vi "Main_NoAndor.vi"() -> ()   [LabVIEW 2014]
doc: "This is the main user interface of the Raman spectroscopy system."
uses:
  C:/Users/light/Desktop/Chuanzhen/Labview/Raman/dll/Thorlabs.MotionControl.Controls.dll
  dll/Thorlabs.MotionControl.Controls.dll
  TypeDef/States.ctl
  TypeDef/StageDeviceOut.ctl
  TypeDef/StageHandleIn.ctl
  <vilib>/Utility/miscctls.llb/LVPoint32TypeDef.ctl
  TypeDef/LaserSpot.ctl
  TypeDef/GalvoInput.ctl
  C:/Users/light/Desktop/Chuanzhen/Labview/Raman/dll/ThorLabs.MotionControl.KCube.DCServoCLI.dll
  dll/ThorLabs.MotionControl.KCube.DCServoCLI.dll
  TypeDef/StageSelect.ctl
  TypeDef/inputImages.ctl
  C:/Users/light/Desktop/Chuanzhen/Labview/Raman/dll/Thorlabs.MotionControl.GenericMotorCLI.dll
  dll/Thorlabs.MotionControl.GenericMotorCLI.dll
panel:
  in  "a2":dbl caption="Offset"
  out "Spot Y":dbl
  out "Spot X":dbl
  in  "Box":cluster{"Width":dbl, " Height":dbl}={"Width"=200.0, " Height"=214.0}
  in  "Galvo Reset":bool
  in  "a1":dbl=8.2 caption="Offset"
  in  "a0":dbl=4.0 caption="Offset"
  in  "Galvo Stop":bool
  out "Total_Frame_Y":dbl
  out "Total_Frame_X":dbl
  out "Frame_Y":dbl
  out "Frame_X":dbl
  in  "Destination":dbl=12.0
  in  "Save Path":path=path "C:/Users/light/Desktop/Chuanzhen/test"
  in  "Scan":bool
  in  "Velocity: X and Y axis":T1(radio)=enum."0.05mm"
  in  "MoveTo":bool
  in  "Jogstep of Z axis":T2(radio)=enum."10step"
  in  "Z axis_d":bool
  in  "Z axis_u":bool
  in  "Y axis_F":bool
  in  "Y axis_B":bool
  out "Y_axis":dbl
  out "X_axis":dbl
  out "Z_axis":dbl
  in  "Reset":bool
  in  "X axis_L":bool
  in  "X axis_R":bool
  in  "Down":bool
  in  "Top":bool
  in  "Right":bool
  in  "Left":bool
  in  "Snap":bool
  out "Boolean":bool
  in  "Pixel Size Y (um)":dbl=0.0877
  in  "LaserSpot":bool
  in  "Pixel Size X (um)":dbl=0.0877
  in  "Aim":bool
  in  "Galvo DC":bool
  out "Sample Rate":dbl=1000.0 format="%0.2f"
  out "Initialization finished":bool
  out "Focal plane (mm)":dbl
  out "Delay (s)":dbl=0.9 format="%#_13g"
  in  "Jog size (um)":dbl=2.0
  out "ZoomRatio":dbl format="%#_2g"
  in  "Focus":bool
  out "Live video":picture caption="600 x 480"
  in  "Next step":bool
  in  "Camera ID":u32
  out "Bits/Pixel":i32=8
  in  "Autogain":bool
  in  "Master Gain":i32(slide) min=0 max=100 scale=0.0..100.0
  in  "Hotpixel correction 2":bool
  in  "Blacklevel compensation":bool
  in  "Edge Filter":i32(ring)=2 items=["High"=1, "Low"=2]
  in  "Edge Filter Enable / Disable":bool
  in  "Exposure time (ms)":dbl(slide)=11.094175438596492 min=0.008982456140350877 max=101.68743859649123 step=0.05487719298245614 scale=0.008982456140350877..101.68743859649123 scale format="%#.3g"
  in  "Pixel clock":i32(slide)=20 min=7 max=86 scale=7.0..86.0
  in  "Frame rate":dbl(slide)=9.827169720568149 min=0.5 max=17.288905497022668 step=5.487719298245614e-05 scale=0.5..17.288905497022668 scale format="%^#_3g"
  in  "Blacklevel Offset":i32(slide) min=0 max=255 scale=0.0..255.0
  out "FPS":dbl=6.258409738085552
  out "Width":i32=640
  out "Height":i32=480
  in  "Stage Control":enum32{"X axis", "Y axis", "Z axis"}(tab)
  in  "X axis":refnum<k24>(container)
  in  "Y axis":refnum<k24>(container)
  in  "Z axis":refnum<k24>(container)
  in  "Quit":bool
  out "Waveform Graph":waveform(dbl)[](graph)=[{"t0"=timestamp(0 s since 1904-01-01), "dt"=0.001, "Y"=[]}]
  # "Camera Control"
  # "Galvo Control"
  # "Objective: CFI Plan Fluor ELWD 60x (1.27 NA) \nThe depth of field: 1.78 um\nPixel Size: 0.0877um/px"
  # "Attention: \ndon't click button very fast"
  # "Auto Focus"
  # "Aim"
  # "Motor Control"
  # "Adjust laser spot lightly"
  # "Stage Scan"
  # "Total_Frame"
  # "Current_Frame"
  # "X"
  # "Y"
  # "Focus distance ia about 2mm"
  # "Stepsize:"
  # "Jogstep:"
  # "0.00003mm/step"
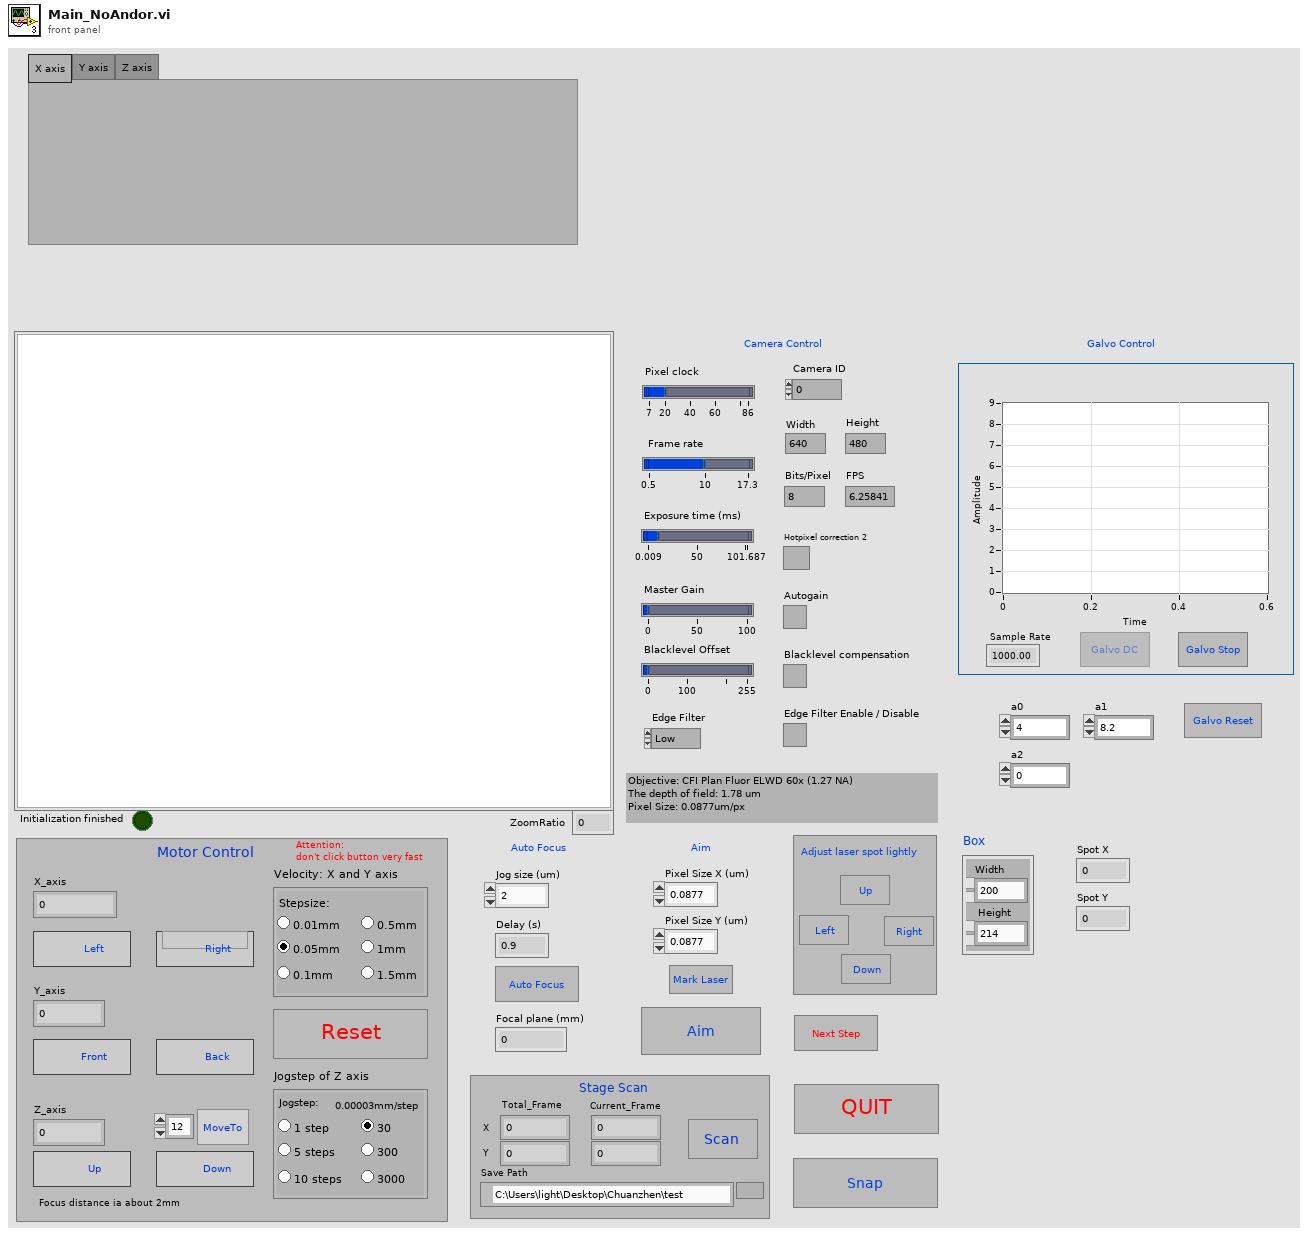
[diagram p1: front panel]
types:
  T1 = enum32{"0.01mm", "0.05mm", "0.1mm", "0.5mm", "1mm", "1.5mm"}
  T2 = enum32{"1step", "2step", "5step", "10step", "15step", "20step"}
  T3 = typedef "LaserSpot.ctl" = cluster{"Laser X":dbl, "Laser Y":dbl}
  T4 = cluster{"left":i16, "top":i16, "right":i16, "bottom":i16}
  T5 = typedef "LVPoint32TypeDef.ctl" = cluster{"Horizontal":i32, "Vertical":i32}
  T6 = typedef "StageHandleIn.ctl" = cluster{"Z StageHandle in":refnum<k24>, "X StageHandle in":refnum<k24>, "Y StageHandle in":refnum<k24>}
  T7 = typedef "StageDeviceOut.ctl" = cluster{"Device Z":refnum<k24>, "Device X":refnum<k24>, "Device Y":refnum<k24>}
  T8 = typedef "States.ctl" = enum16{"Initialize", "CMOS live", "Shut down"}
  T9 = enum8{"Enabled", "Disabled", "Disabled and Grayed Out"}
  T10 = typedef "GalvoInput.ctl" = cluster{"Sample Rate":dbl, "Sample Clock Source":tag, "Max Voltage":dbl, "Min Voltage":dbl, "Physical Channel(s)":tag}
  T11 = cluster{"Width":u16, "Style":enum32{"Solid", "Dash", "Dot", "DashDot", "DashDotDot"}}
  T12 = typedef "StageSelect.ctl" = enum16{"X axis", "Y axis", "Z axis"}
  T13 = typedef "inputImages.ctl" = cluster{"Image2":u8[][], "Image3":u8[][], "Image4":u8[][], "Image1":u8[][]}
  T14 = typedef "StageHandleOut.ctl" = cluster{"Z StageHandle out":refnum<k24>, "X StageHandle out":refnum<k24>, "Y StageHandle out":refnum<k24>}
  T15 = typedef "LVBoundsTypeDef.ctl" = cluster{"Width":u32, "Height":u32}
  T16 = typedef "imagedata.ctl" = cluster{"image type":i32, "image depth":i32, "image":u8[], "mask":u8[], "colors":u32[], "Rectangle":cluster{"left":i16, "top":i16, "right":i16, "bottom":i16}}
  T17 = typedef "LVPositionTypeDef.ctl" = cluster{"Left":i32, "Top":i32}
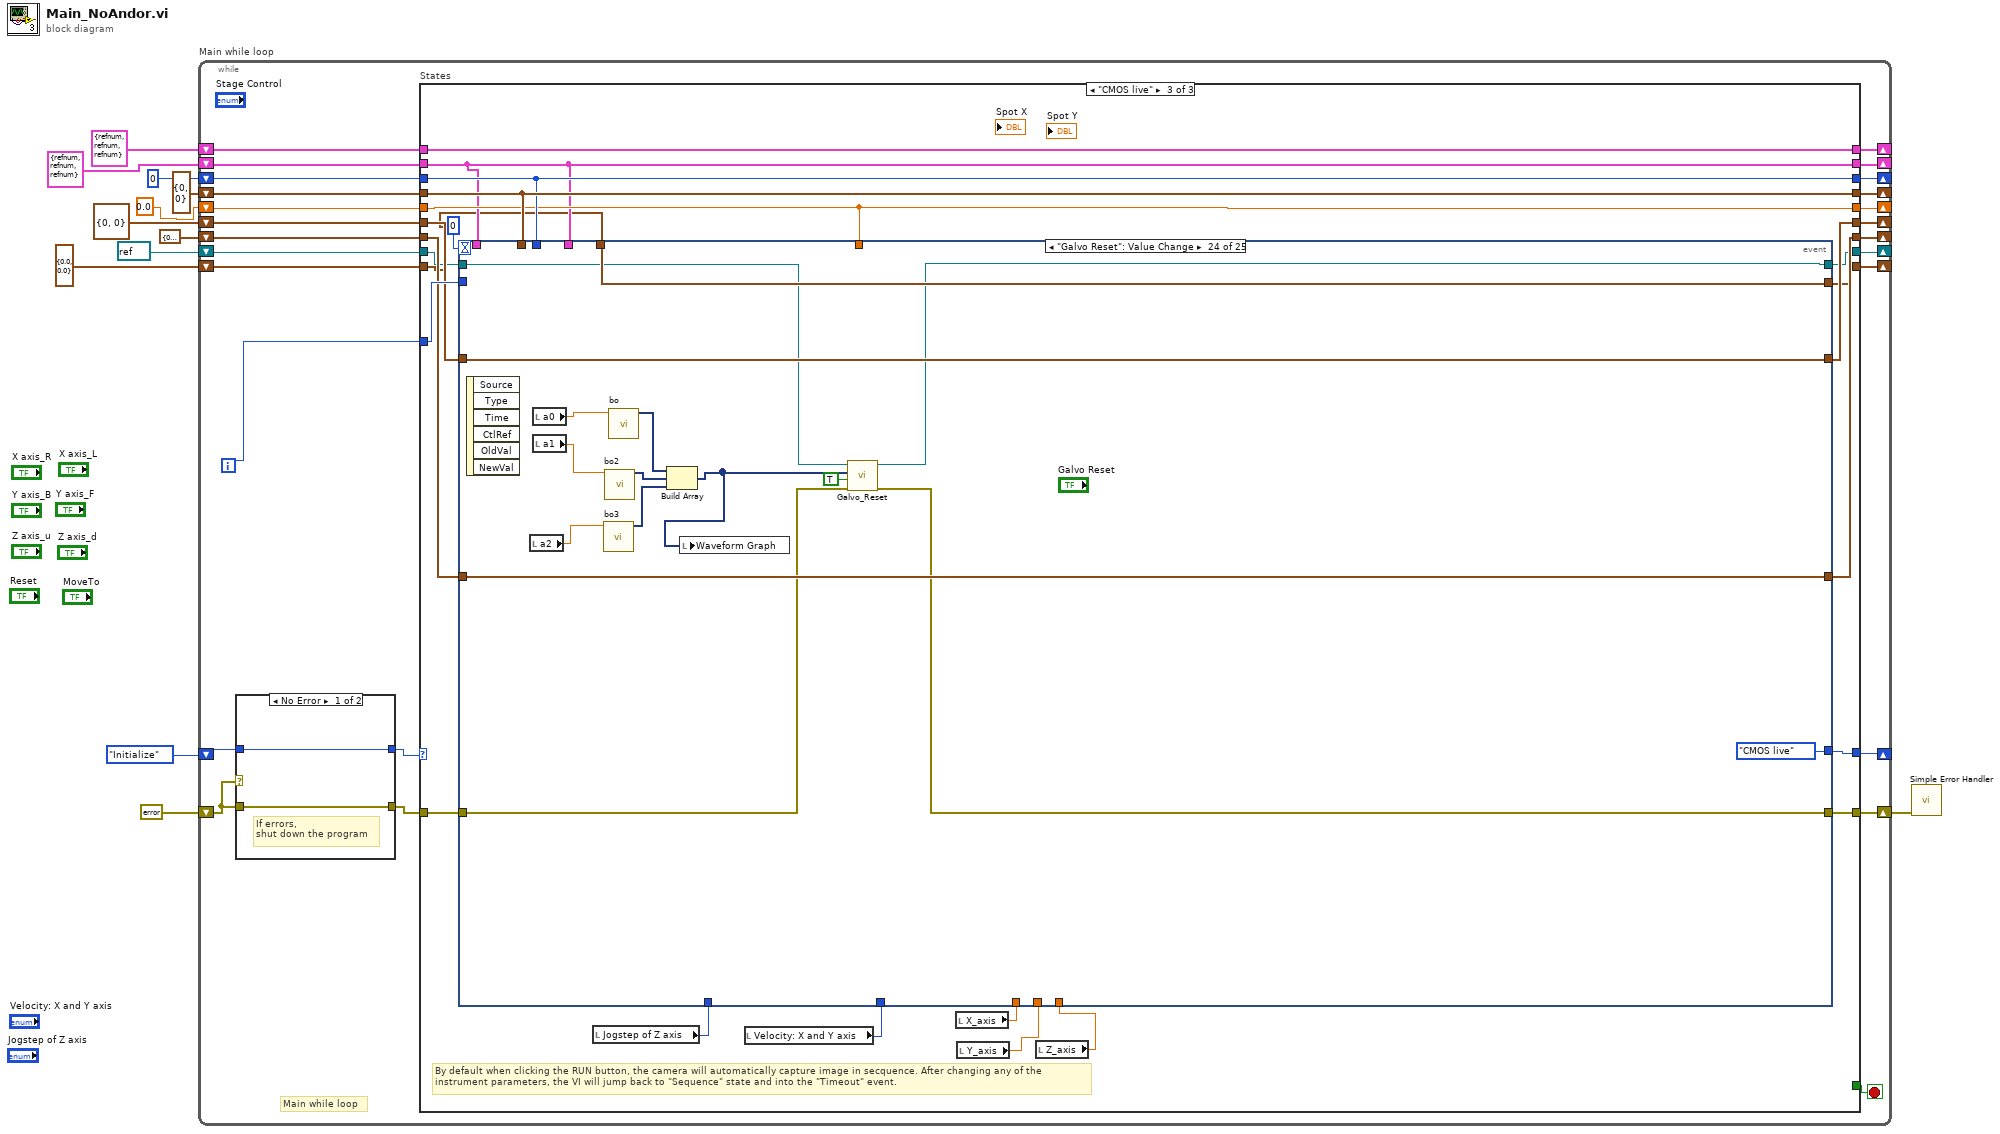
[diagram p0: block diagram]
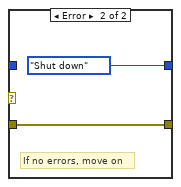
[diagram p2: hidden frame]
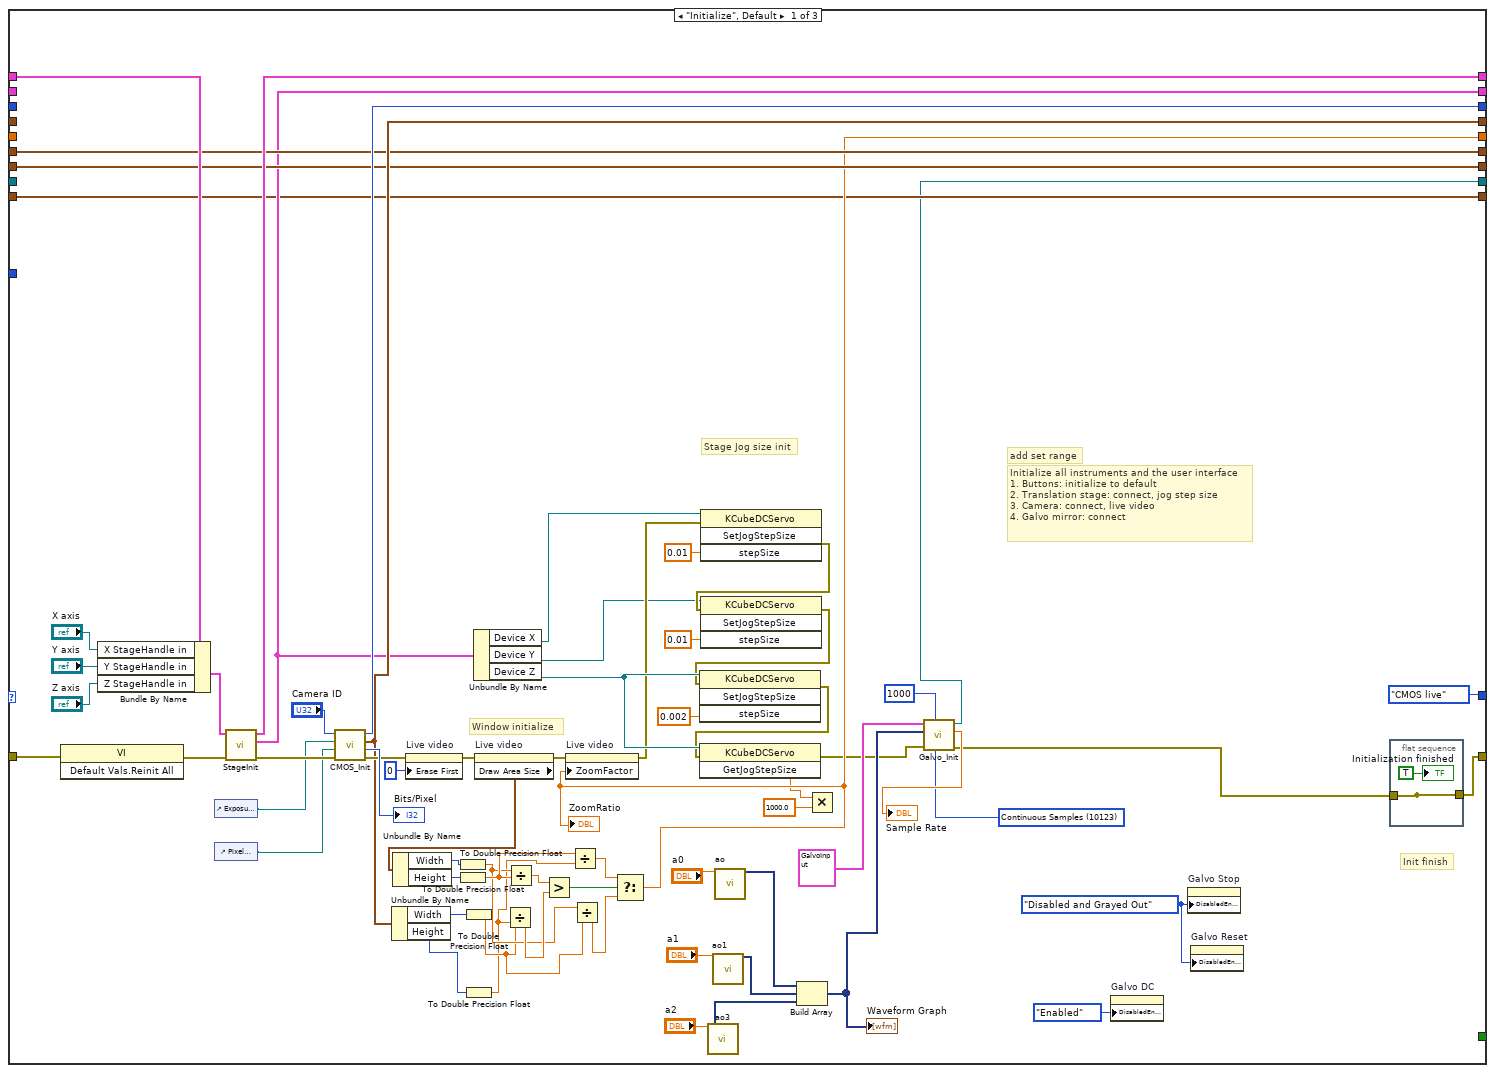
[diagram p3: hidden frame]
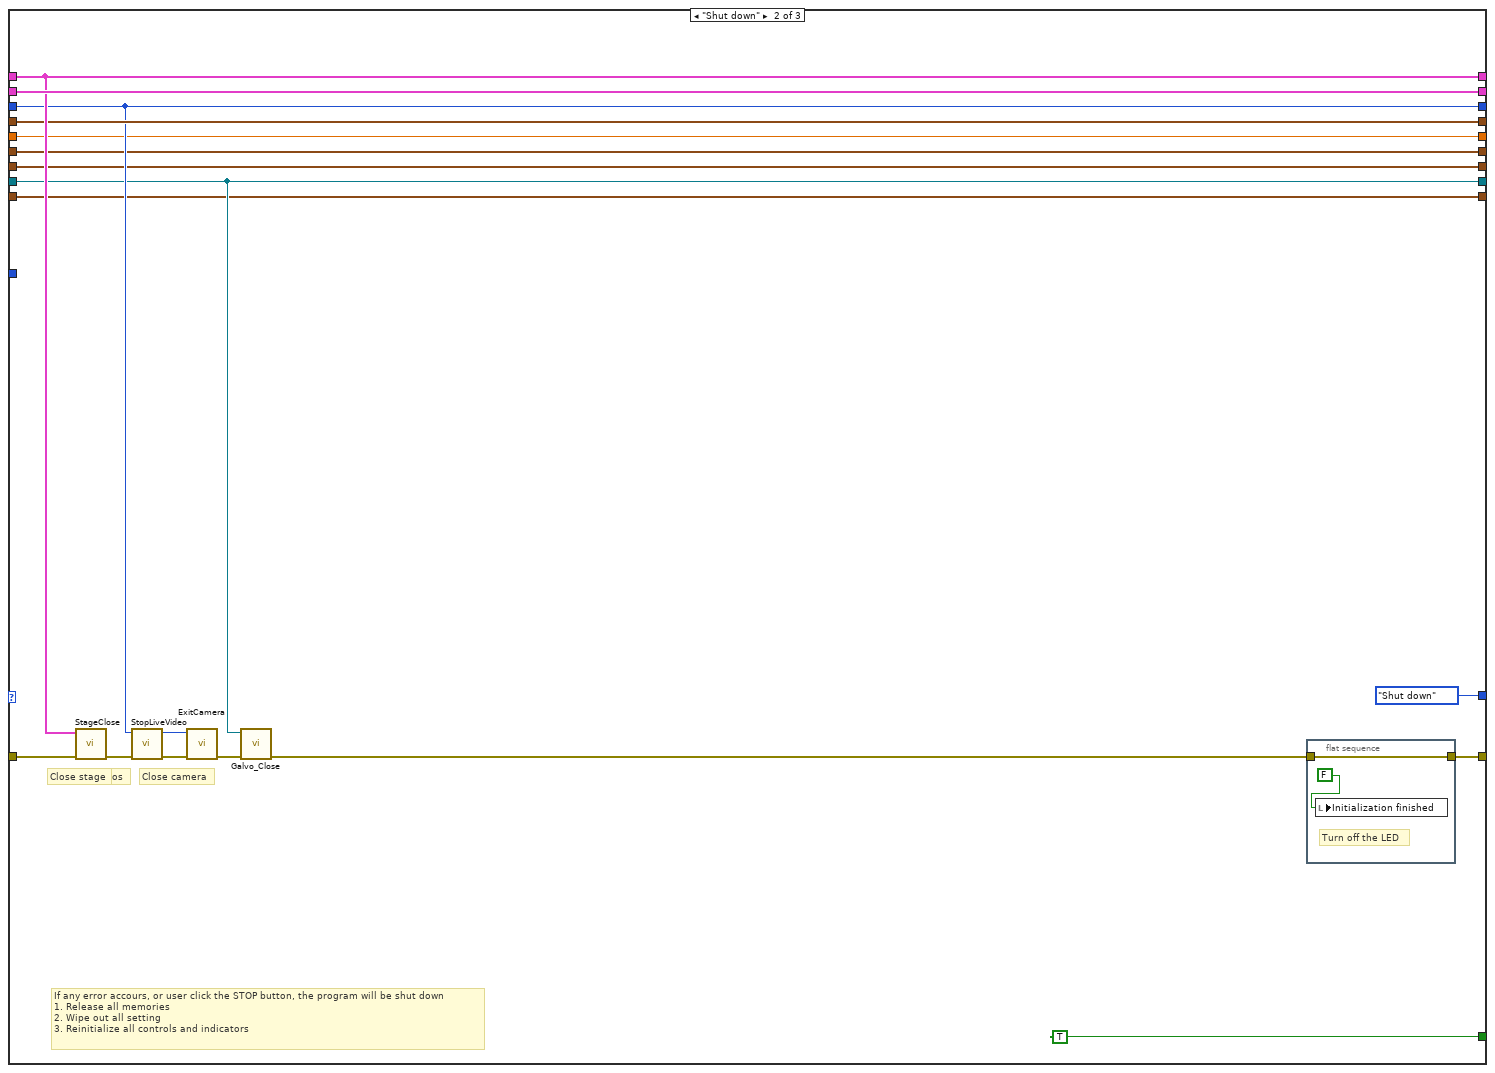
[diagram p4: hidden frame]
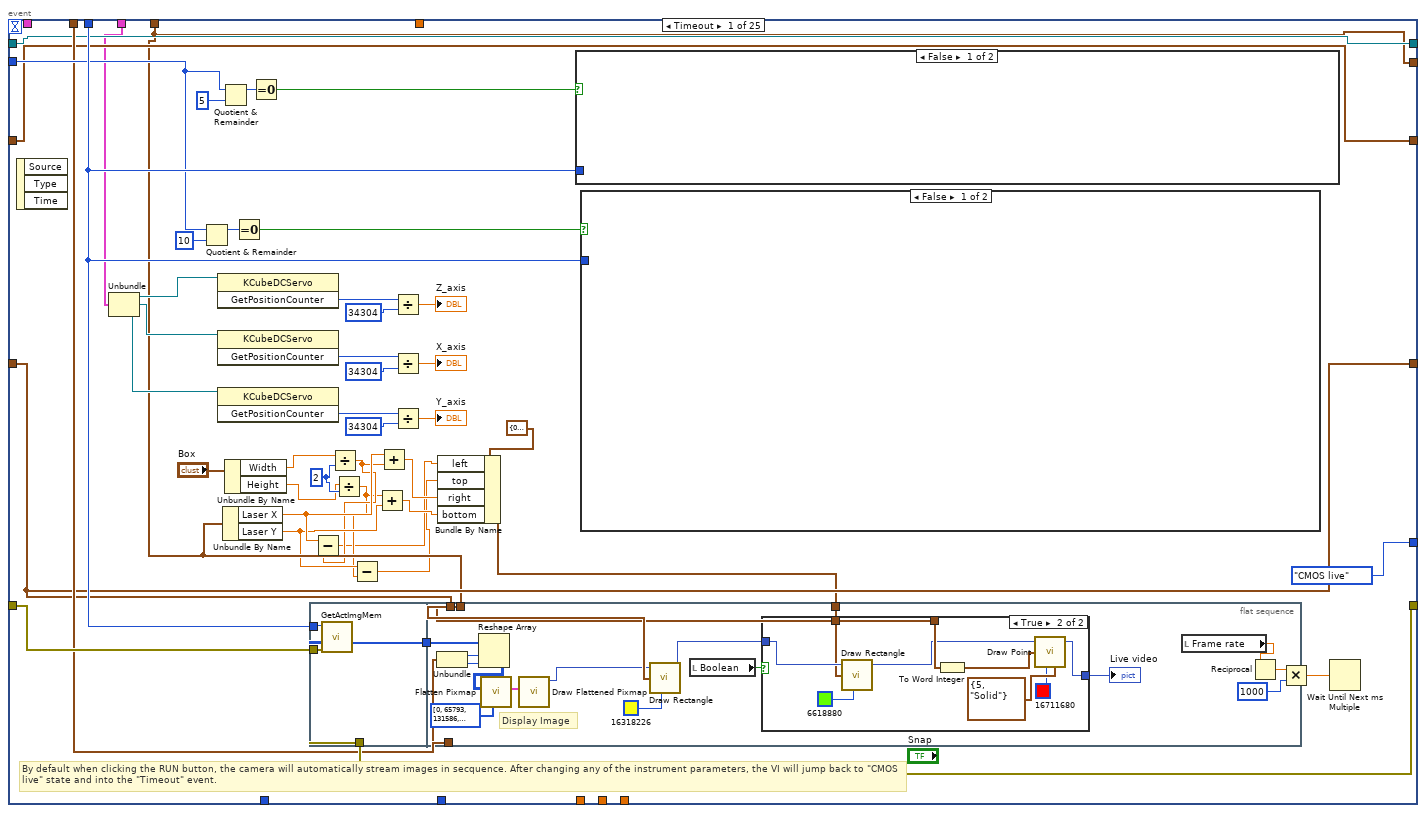
[diagram p5: hidden frame]
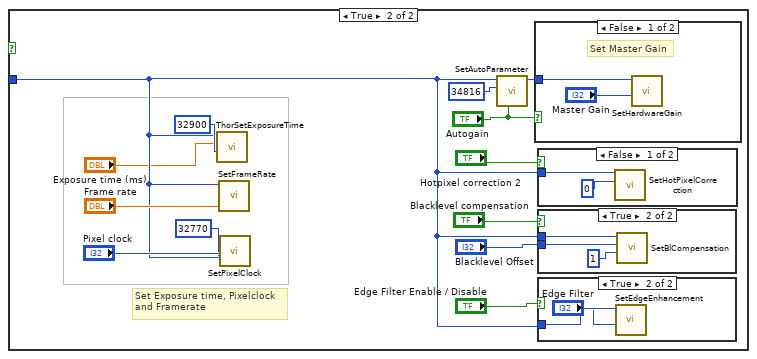
[diagram p6: hidden frame]
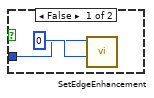
[diagram p7: hidden frame]
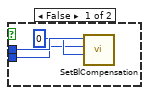
[diagram p8: hidden frame]
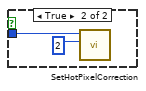
[diagram p9: hidden frame]
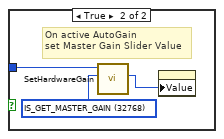
[diagram p10: hidden frame]
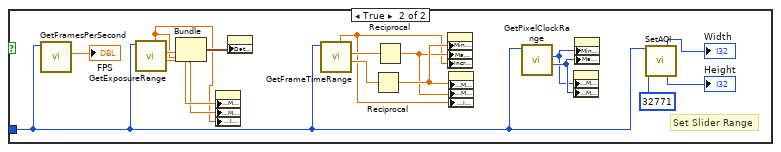
[diagram p11: hidden frame]
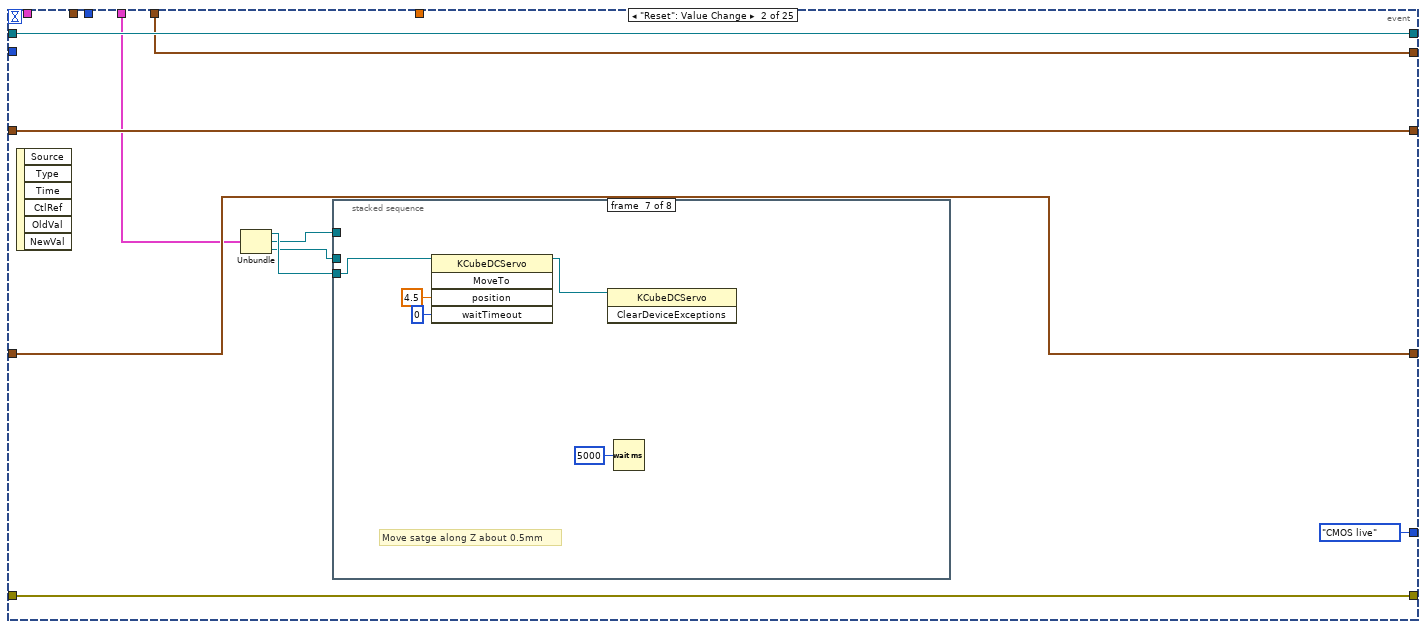
[diagram p13: hidden frame]
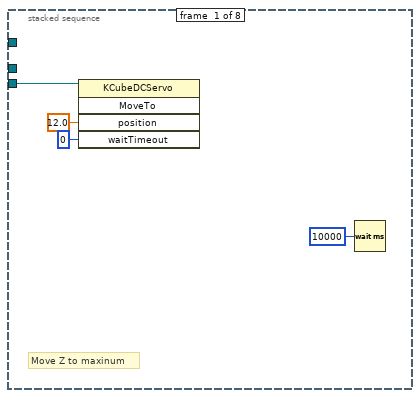
[diagram p14: hidden frame]
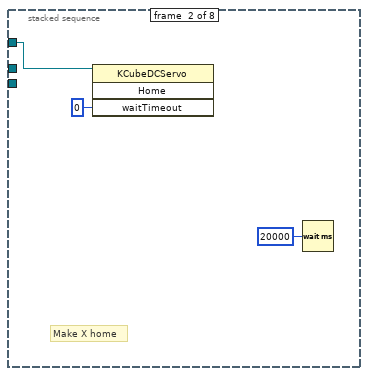
[diagram p15: hidden frame]
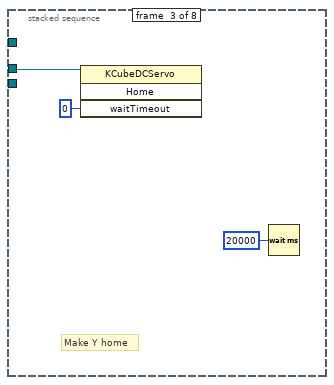
[diagram p16: hidden frame]
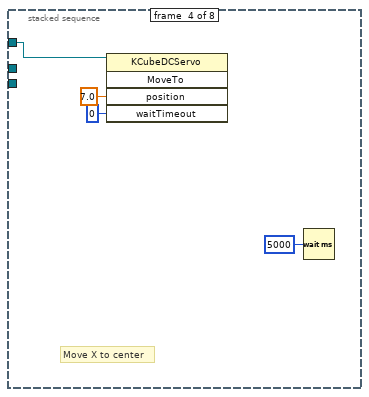
[diagram p17: hidden frame]
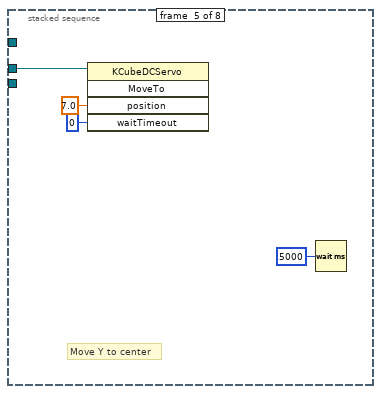
[diagram p18: hidden frame]
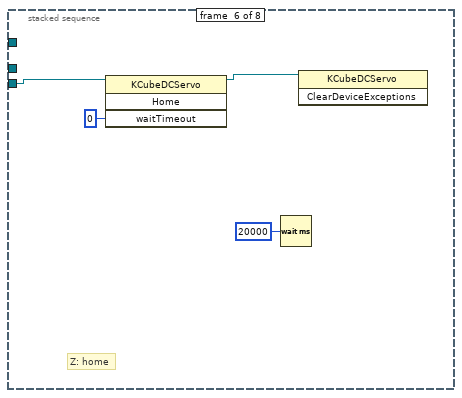
[diagram p19: hidden frame]
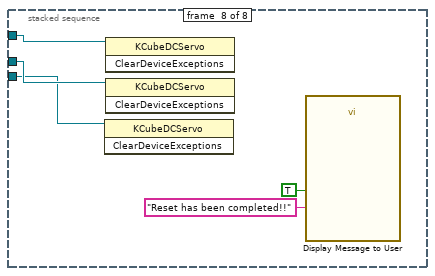
[diagram p20: hidden frame]
diagram:
  n1 = while "Main while loop" {
    shift-right: [w33] -> _
    shift-left: States."Initialize" -> [w38]
    shift-right: [w36] -> w10
    shift-left: errorcluster {"status"=FALSE, "code"=0, "source"=""} ("error out") -> [w32]
    shift-right: [w30] -> _
    shift-left: T6 {"Z StageHandle in"=refnum, "X StageHandle in"=refnum, "Y StageHandle in"=refnum} ("StageHandle In") -> [w31]
    shift-right: [w29] -> _
    shift-left: T7 {"Device Z"=refnum, "Device X"=refnum, "Device Y"=refnum} ("Device Out") -> [w28]
    shift-right: [w27] -> _
    shift-left: u32 0 ("CMOS Handle Out") -> [w26]
    shift-right: [w24] -> _
    shift-left: cluster{"Height":i32, "Width":i32} {"Height"=0, "Width"=0} ("WidthAndHeight") -> [w23]
    shift-right: [w22] -> _
    shift-left: 0.0 -> [w17]
    shift-right: [w21] -> _
    shift-left: T5 {"Horizontal"=0, "Vertical"=0} ("Coords") -> [w20]
    shift-right: [w19] -> _
    shift-left: T4 {"left"=0, "top"=0, "right"=0, "bottom"=0} ("rect") -> [w18]
    shift-right: [w16] -> _
    shift-left: refnum<k21> refnum ("task out") -> [w15]
    shift-right: [w14] -> _
    shift-left: T3 {"Laser X"=0.0, "Laser Y"=0.0} ("LaserSpot 2") -> [w13]
    i -> [w25]
    stop <- w34 stop-if-true
    # "Main while loop"
    n2 = case shown="No Error" w32 {
      tunnel: w32 -> [w40 w42]
      tunnel: [w40 w42] -> w35
      tunnel: w38 -> [w39 _]
      tunnel: [w39 States."Shut down"] -> w37
      frame No Error {
        # "If errors,\nshut down the program"
      }
      frame Error {
        # "If no errors, move on"
      }
    }
    n3 = case "States" shown="\"CMOS live\"" w37 {
      tunnel: [w53 w117 w152] -> w36
      tunnel: w35 -> [w109 w127 w153]
      tunnel: [_ TRUE _] -> w34
      tunnel: [States."CMOS live" States."Shut down" w154] -> w33
      tunnel: w31 -> [w107 w126 w155]
      tunnel: [w106 w126 w155] -> w30
      tunnel: [w73 w128 w142] -> w29
      tunnel: w28 -> [_ w128 w142]
      tunnel: [w100 w121 w148] -> w27
      tunnel: w26 -> [_ w121 w148]
      tunnel: w25 -> [_ _ w150]
      tunnel: [w81 w125 w149] -> w24
      tunnel: w23 -> [_ w125 w149]
      tunnel: [w74 w120 w143] -> w22
      tunnel: w17 -> [_ w120 w143]
      tunnel: [w76 w119 w147] -> w21
      tunnel: w20 -> [w76 w119 w146]
      tunnel: [w75 w118 w145] -> w19
      tunnel: w18 -> [w75 w118 w144]
      tunnel: [w54 w115 w140] -> w16
      tunnel: w15 -> [_ w115 w141]
      tunnel: [w59 w113 w139] -> w14
      tunnel: w13 -> [w59 w113 w138]
      frame "Initialize", Default {
        w45 = 10123 items=["Finite Samples"=10178, "Continuous Samples"=10123, "Hardware Timed Single Point"=12522] ("Sample Mode")
        w47 = T9."Disabled and Grayed Out" ("Disabled")
        # "Init finish"
        # "add set range"
        # "Stage Jog size init"
        # "Window initialize"
        # "Initialize all instruments and the user interface\n1. Buttons: initialize to default\n2. Translation stage: connect, jog step size\n3. Camera: connect, live video\n4. Galvo mirror: connect"
        n4 = invoke class="VI" method="Default Vals.Reinit All"(error in=w109) -> (error out=w108:errorcluster)  [unwired: 2 in, 2 out]
        n5 = Bundle By Name(cluster=w107, "X StageHandle in"="X axis", "Y StageHandle in"="Y axis", "Z StageHandle in"="Z axis") -> (w105:T6)
        n6 = control-ref of="Exposure time (ms)"() -> (w99:refnum<vi>)
        n7 = control-ref of="Pixel clock"() -> (w98:refnum<vi>)
        n8 = call "StageInit.vi"("error in (no error)"=w108, "StageHandle In"=w105) -> ("error out"=w101:errorcluster, "Device Out"=w73:T7, "StageHandle Out"=w106:T14)  [unwired: 7 in]
        n9 = call "CMOS_Init.vi"("error in"=w101, "Pixel clock"=w98, "Exposure time"=w99, "Camera ID"="Camera ID") -> ("error out"=w95:errorcluster, "Bits/Pixel"=→"Bits/Pixel":i32, "WidthAndHeight"=w81:cluster{"Height":i32, "Width":i32}, "CMOS Handle Out"=w100:u32)  [unwired: 3 in]
        n10 = Unbundle By Name(w81) -> ("Width"=w80:i32, "Height"=w79:i32)
        n11 = property on="Live video" class="Pict"(error in=w95, "Erase First"=u8 0) -> (error out=w83:errorcluster)  [unwired: 1 in, 1 out]
        n12 = To Double Precision Float(number=w80) -> (double precision float=w78:dbl)
        n13 = To Double Precision Float(number=w79) -> (double precision float=w77:dbl)
        n14 = Unbundle By Name(w73) -> ("Device X"=w62:refnum<k24>, "Device Y"=w61:refnum<k24>, "Device Z"=w71:refnum<k24>)
        n15 = property on="Live video" class="Pict"(error in=w83) -> (error out=w82:errorcluster, "Draw Area Size"=w93:T15)  [unwired: 1 in, 1 out]
        n16 = Unbundle By Name(w93) -> ("Width"=w91:u32, "Height"=w92:u32)
        n17 = To Double Precision Float(number=w91) -> (double precision float=w85:dbl)
        n18 = To Double Precision Float(number=w92) -> (double precision float=w87:dbl)
        n19 = Divide(x=w78, y=w77) -> (x/y=w88:dbl)
        n20 = Divide(x=w85, y=w87) -> (x/y=w90:dbl)
        n21 = Greater?(x=w90, y=w88) -> (0:w89:bool)
        n22 = Divide(x=w87, y=w77) -> (x/y=w86:dbl)
        n23 = Divide(x=w85, y=w78) -> (x/y=w84:dbl)
        n24 = Select(t=w86, s=w89, f=w84) -> (s? t:f=w74:dbl)
        "ZoomRatio" <- w74
        n25 = property on="Live video" class="Pict"(error in=w82, "ZoomFactor"=w74) -> (error out=w65:errorcluster)  [unwired: 1 in, 1 out]
        n26 = invoke class="KCubeDCServo" method="SetJogStepSize"(reference=w62, error in=w65, "stepSize"=0.01) -> (error out=w64:errorcluster)  [unwired: 1 in, 3 out]
        n27 = invoke class="KCubeDCServo" method="SetJogStepSize"(reference=w61, error in=w64, "stepSize"=0.01) -> (error out=w63:errorcluster)  [unwired: 1 in, 3 out]
        n28 = invoke class="KCubeDCServo" method="SetJogStepSize"(reference=w71, error in=w63, "stepSize"=0.002) -> (error out=w70:errorcluster)  [unwired: 1 in, 3 out]
        n29 = invoke class="KCubeDCServo" method="GetJogStepSize"(reference=w71, error in=w70) -> (error out=w56:errorcluster, "GetJogStepSize"=w69:dbl)  [unwired: 1 in, 1 out]
        n30 = call "ao3"("Offset"="a2") -> ("DC"=w60:dynamicdata)  [unwired: 13 in, 1 out]
        n31 = call "ao1"("Offset"="a1") -> ("DC"=w50:dynamicdata)  [unwired: 13 in, 1 out]
        n32 = call "ao"("Offset"="a0") -> ("DC"=w49:dynamicdata)  [unwired: 13 in, 1 out]
        n33 = Build Array(w49, w50, w60) -> (w57:dynamicdata[])
        "Waveform Graph" <- w57
        n34 = Multiply(x=w69, y=1000.0) -> ()  [unwired: 1 out]
        n35 = call "Galvo_Init.vi"("Sample Mode"=w45, "samples per channel"=1000, "error in"=w56, "Signal array"=w57, "Galvo_Input"=T10 {"Sample Rate"=1000.0, "Sample Clock Source"="OnboardClock", "Max Voltage"=10.0, "Min Voltage"=-10.0, "Physical Channel(s)"="Dev1/ao0,Dev1/ao1,Dev1/ao3"} ("Galvo1_1")) -> ("error out"=w48:errorcluster, "Actual Sample Rate"=→"Sample Rate":dbl, "task out"=w54:refnum<k21>)  [unwired: 4 in]
        n36 = property on="Galvo DC" class="Bool"("DisabledEnum"=T9."Enabled" ("Disabled")) -> ()  [unwired: 2 in, 2 out]
        n37 = property on="Galvo Stop" class="Bool"("DisabledEnum"=w47) -> ()  [unwired: 2 in, 2 out]
        n38 = property on="Galvo Reset" class="Bool"("DisabledEnum"=w47) -> ()  [unwired: 2 in, 2 out]
        n39 = flat-sequence {
          tunnel: [w111] -> _
          tunnel: w48 -> [w111]
          tunnel: [w111] -> w53
          frame #0 {
            "Initialization finished" <- TRUE ("Initialization finished")
          }
        }
      }
      frame "Shut down" {
        # "Close 3 galvos"
        # "Close camera"
        # "Close stage"
        # "If any error accours, or user click the STOP button, the program will be shut down\n1. Release all memories\n2. Wipe out all setting\n3. Reinitialize all controls and indicators"
        n40 = call "StageClose.vi"("error in (no error)"=w127, "StageHandle In"=w126) -> ("error out"=w124:errorcluster)  [unwired: 9 in]
        n41 = call "StopLiveVideo.vi"("error in"=w124, "Camera Handle In"=w121) -> ("error out"=w123:errorcluster, "Camera Handle Out"=w122:u32)  [unwired: 8 in]
        n42 = call "ExitCamera.vi"("error in"=w123, "Camera Handle In"=w122) -> ("error out"=w116:errorcluster)  [unwired: 9 in]
        n43 = call "Galvo_Close.vi"("error in"=w116, "task/channels in"=w115) -> ("error out"=w114:errorcluster)  [unwired: 9 in]
        n44 = flat-sequence {
          tunnel: w114 -> [w132]
          tunnel: [w132] -> w117
          frame #0 {
            # "Turn off the LED"
            n45 = local write "Initialization finished"(FALSE ("Initialization finished")) -> ()
          }
        }
      }
      frame "CMOS live" {
        # "By default when clicking the RUN button, the camera will automatically capture image in secquence. After changing any of the \ninstrument parameters, the VI will jump back to \"Sequence\" state and into the \"Timeout\" event."
        n46 = local read "Jogstep of Z axis"() -> (w133:T2)
        n47 = local read "Velocity: X and Y axis"() -> (w137:T1)
        n48 = local read "X_axis"() -> (w136:dbl)
        n49 = local read "Y_axis"() -> (w135:dbl)
        n50 = local read "Z_axis"() -> (w134:dbl)
        n51 = event shown="[23] \"Galvo Reset\": Value Change" {
          selector: _ -> [_ _ _ _ _ _ _ _ _ _ _ _ _ _ _ _ _ _ _ _ _ _ _ _ _]
          dyn-events: _ -> [_ _ _ _ _ _ _ _ _ _ _ _ _ _ _ _ _ _ _ _ _ _ _ _ _]
          timeout: 0 -> [_ _ _ _ _ _ _ _ _ _ _ _ _ _ _ _ _ _ _ _ _ _ _ _ _]
          tunnel: [States."CMOS live" States."CMOS live" States."CMOS live" States."CMOS live" States."CMOS live" States."CMOS live" States."CMOS live" States."CMOS live" States."CMOS live" States."CMOS live" States."CMOS live" States."Shut down" States."CMOS live" States."CMOS live" States."Shut down" States."CMOS live" States."CMOS live" States."CMOS live" States."CMOS live" States."CMOS live" States."CMOS live" States."CMOS live" States."CMOS live" States."CMOS live" States."CMOS live"] -> w154
          tunnel: w153 -> [w192 w290 w328 w597 w620 w645 w668 w693 w717 w737 w738 w756 w760 w768 w800 w847 w917 w939 w950 w961 w972 w983 w988 w1003 w1013]
          tunnel: [w191 w290 w327 w597 w620 w645 w668 w693 w717 w737 w738 w756 w760 w768 w800 w819 w918 w939 w950 w961 w972 w983 w987 w1002 w1014] -> w152
          tunnel: w148 -> [w190 _ w326 _ _ _ _ _ _ _ w747 _ _ _ _ w844 _ _ _ _ _ _ _ _ _]
          tunnel: w150 -> [w189 _ _ _ _ _ _ _ _ _ _ _ _ _ _ _ _ _ _ _ _ _ _ _ _]
          tunnel: w149 -> [w188 _ w325 _ _ _ _ _ _ _ w740 _ _ _ _ w843 _ _ _ _ _ _ _ _ _]
          tunnel: [w186 w289 w337 w596 w619 w644 w667 w692 w716 w736 w751 w755 w762 w770 w799 w849 w921 w938 w949 w960 w971 w982 w993 w1009 w1019] -> w147
          tunnel: w146 -> [w186 w289 w337 w596 w619 w644 w667 w692 w716 w736 w751 w755 _ w770 w799 w849 w921 w938 w949 w960 w971 w982 w993 w1009 w1019]
          tunnel: [w187 w288 w323 w595 w618 w643 w666 w691 w715 w735 w750 w754 w761 w773 w798 w842 w916 w927 w948 w959 w970 w981 w992 w1008 w1018] -> w145
          tunnel: w144 -> [w187 w288 w323 w595 w618 w643 w666 w691 w715 w735 w750 w754 w761 _ w798 w842 w916 w927 w948 w959 w970 w981 w992 w1008 w1018]
          tunnel: w143 -> [_ _ _ _ _ _ _ _ _ _ _ _ _ w772 _ _ _ _ _ _ _ _ _ _ _]
          tunnel: w142 -> [_ _ _ _ _ _ _ _ _ _ _ _ _ _ _ w818 _ _ _ _ _ _ _ _ _]
          tunnel: w142 -> [w183 w284 w329 w592 w614 w637 w661 w684 w709 w728 _ _ _ _ _ w840 w905 _ _ _ _ _ _ _ _]
          tunnel: [w185 w287 w336 w594 w617 w642 w665 w690 w714 w734 w749 w753 w759 w767 w797 w803 w920 w937 w947 w958 w969 w980 w990 w1004 w1012] -> w140
          tunnel: w141 -> [w185 w287 w336 w594 w617 w642 w665 w690 w714 w734 w749 w753 w759 w767 w797 w803 w920 w937 w947 w958 w969 w980 w989 w1005 w1015]
          tunnel: [w168 w286 w334 w593 w616 w641 w664 w689 w713 w733 w748 w752 w758 w766 w796 w802 w882 w925 w944 w953 w965 w976 w986 w1007 w1017] -> w139
          tunnel: w138 -> [w168 w286 w334 w593 w616 w641 w664 w689 w713 w733 w748 w752 w758 w766 w796 w802 w882 _ w943 w954 w966 w977 w986 w1007 w1017]
          tunnel: w137 -> [_ _ _ w584 w609 w632 w657 _ _ _ _ _ _ _ _ _ _ _ _ _ _ _ _ _ _]
          tunnel: w136 -> [_ _ _ w587 w612 _ _ _ _ _ _ _ _ _ _ _ _ _ _ _ _ _ _ _ _]
          tunnel: w135 -> [_ _ _ _ _ w634 w659 _ _ _ _ _ _ _ _ _ _ _ _ _ _ _ _ _ _]
          tunnel: w134 -> [_ _ _ _ _ _ _ w681 w705 _ _ _ _ _ _ _ _ _ _ _ _ _ _ _ _]
          tunnel: w133 -> [_ _ _ _ _ _ _ w685 w708 _ _ _ _ _ _ _ _ _ _ _ _ _ _ _ _]
          event Timeout {
            w167 = 2
            # "By default when clicking the RUN button, the camera will automatically stream images in secquence. After changing any of the instrument parameters, the VI will jump back to \"CMOS live\" state and into the \"Timeout\" event."
            n52 = event-data() -> ()  [unwired: 1 in, 3 out]
            n53 = Unbundle(w183) -> ("Device Z"=w173:refnum<k24>, "Device X"=w172:refnum<k24>, "Device Y"=w171:refnum<k24>)
            n54 = Quotient & Remainder(x=w189, y=10) -> (x-y*floor(x/y)=w199:i32)  [unwired: 1 out]
            n55 = invoke class="KCubeDCServo" method="GetPositionCounter"(reference=w173) -> ("GetPositionCounter"=w182:i32)  [unwired: 2 in, 2 out]
            n56 = invoke class="KCubeDCServo" method="GetPositionCounter"(reference=w172) -> ("GetPositionCounter"=w181:i32)  [unwired: 2 in, 2 out]
            n57 = invoke class="KCubeDCServo" method="GetPositionCounter"(reference=w171) -> ("GetPositionCounter"=w180:i32)  [unwired: 2 in, 2 out]
            n58 = Quotient & Remainder(x=w189, y=5) -> (x-y*floor(x/y)=w202:i32)  [unwired: 1 out]
            n59 = Unbundle By Name(w168) -> ("Laser X"=w162:dbl, "Laser Y"=w161:dbl)
            n60 = Unbundle By Name("Box") -> ("Width"=w166:dbl, "Height"=w165:dbl)
            n61 = Equal To 0?(x=w199) -> (x = 0?=w197:bool)
            n62 = Equal To 0?(x=w202) -> (x = 0?=w201:bool)
            n63 = flat-sequence {
              tunnel: [w254] -> w203
              tunnel: w190 -> [w255]
              tunnel: w192 -> [w253]
              tunnel: [w252] -> w191
              tunnel: w203 -> [w270]
              tunnel: w188 -> [w269]
              tunnel: w187 -> [w262]
              tunnel: w168 -> [w258]
              tunnel: w156 -> [w256]
              frame #0 {
                n64 = call "GetActImgMem.vi"("error in"=w253, "Camera Handle In"=w255) -> ("error out"=w252:errorcluster, "Image Memory Out"=w254:u8[])  [unwired: 6 in, 2 out]
              }
              frame #1 {
                # "Display Image"
                n65 = Unbundle(w269) -> ("Height"=w268:i32, "Width"=w267:i32)
                n66 = Reshape Array(w270, w268, w267) -> (w266:u8[][])
                n67 = call <vilib>:"Flatten Pixmap.vi"("colors"=u32[] [0, 65793, 131586, 197379, 263172, 328965, 394758, 460551, 526344, 592137, 657930, 723723, 789516, 855309, 921102, 986895, 1052688, 1118481, 1184274, 1250067, 1315860, 1381653, 1447446, 1513239, 1579032, 1644825, 1710618, 1776411, 1842204, 1907997, 1973790, 2039583, 2105376, 2171169, 2236962, 2302755, 2368548, 2434341, 2500134, 2565927, 2631720, 2697513, 2763306, 2829099, 2894892, 2960685, 3026478, 3092271, 3158064, 3223857, 3289650, 3355443, 3421236, 3487029, 3552822, 3618615, 3684408, 3750201, 3815994, 3881787, 3947580, 4013373, 4079166, 4144959, 4210752, 4276545, 4342338, 4408131, 4473924, 4539717, 4605510, 4671303, 4737096, 4802889, 4868682, 4934475, 5000268, 5066061, 5131854, 5197647, 5263440, 5329233, 5395026, 5460819, 5526612, 5592405, 5658198, 5723991, 5789784, 5855577, 5921370, 5987163, 6052956, 6118749, 6184542, 6250335, 6316128, 6381921, 6447714, 6513507, 6579300, 6645093, 6710886, 6776679, 6842472, 6908265, 6974058, 7039851, 7105644, 7171437, 7237230, 7303023, 7368816, 7434609, 7500402, 7566195, 7631988, 7697781, 7763574, 7829367, 7895160, 7960953, 8026746, 8092539, 8158332, 8224125, 8289918, 8355711, 8421504, 8487297, 8553090, 8618883, 8684676, 8750469, 8816262, 8882055, 8947848, 9013641, 9079434, 9145227, 9211020, 9276813, 9342606, 9408399, 9474192, 9539985, 9605778, 9671571, 9737364, 9803157, 9868950, 9934743, 10000536, 10066329, 10132122, 10197915, 10263708, 10329501, 10395294, 10461087, 10526880, 10592673, 10658466, 10724259, 10790052, 10855845, 10921638, 10987431, 11053224, 11119017, 11184810, 11250603, 11316396, 11382189, 11447982, 11513775, 11579568, 11645361, 11711154, 11776947, 11842740, 11908533, 11974326, 12040119, 12105912, 12171705, 12237498, 12303291, 12369084, 12434877, 12500670, 12566463, 12632256, 12698049, 12763842, 12829635, 12895428, 12961221, 13027014, 13092807, 13158600, 13224393, 13290186, 13355979, 13421772, 13487565, 13553358, 13619151, 13684944, 13750737, 13816530, 13882323, 13948116, 14013909, 14079702, 14145495, 14211288, 14277081, 14342874, 14408667, 14474460, 14540253, 14606046, 14671839, 14737632, 14803425, 14869218, 14935011, 15000804, 15066597, 15132390, 15198183, 15263976, 15329769, 15395562, 15461355, 15527148, 15592941, 15658734, 15724527, 15790320, 15856113, 15921906, 15987699, 16053492, 16119285, 16185078, 16250871, 16316664, 16382457, 16448250, 16514043, 16579836, 16645629, 16711422, 0] ("output array 2"), "8-bit pixmap"=w266) -> ("image data"=w265:T16)  [unwired: 9 in]
                n68 = call <vilib>:"Draw Flattened Pixmap.vi"("image data"=w265) -> ("new picture"=w257:picture)  [unwired: 8 in]
                n69 = call <vilib>:"Draw Rectangle.vi"("picture"=w257, "rect"=w262, "color(black)"=u32 16318226) -> ("new picture"=w261:picture)  [unwired: 6 in]
                n70 = local read "Boolean"() -> (w259:bool)
                n71 = case shown="True" w259 {
                  tunnel: w261 -> [w271 w275]
                  tunnel: [w271 w277] -> w260
                  tunnel: w258 -> [_ w276]
                  tunnel: w256 -> [_ w273]
                  frame False {
                  }
                  frame True {
                    n72 = call <vilib>:"Draw Rectangle.vi"("picture"=w275, "rect"=w273, "color(black)"=u32 6618880) -> ("new picture"=w274:picture)  [unwired: 6 in]
                    n73 = To Word Integer(number=w276) -> (16bit integer=w278:cluster{"Laser X":i16, "Laser Y":i16})
                    n74 = call <vilib>:"Draw Point.vi"("picture"=w274, "point(x,y)"=w278, "color(black)"=u32 16711680, "pen"=T11 {"Width"=5, "Style"=enum."Solid"}) -> ("new picture"=w277:picture)  [unwired: 5 in]
                  }
                }
                "Live video" <- w260
              }
            }
            n75 = Divide(x=w166, y=w167) -> (x/y=w160:dbl)
            n76 = Subtract(x=w162, y=w160) -> (x-y=w158:dbl)
            n77 = Divide(x=w165, y=w167) -> (x/y=w159:dbl)
            n78 = Subtract(x=w161, y=w159) -> (x-y=w157:dbl)
            n79 = Add(x=w159, y=w161) -> (x+y=w163:dbl)
            n80 = Add(x=w162, y=w160) -> (x+y=w164:dbl)
            n81 = Divide(x=w182, y=34304) -> (x/y=→"Z_axis":dbl)
            n82 = Divide(x=w181, y=34304) -> (x/y=→"X_axis":dbl)
            n83 = Divide(x=w180, y=34304) -> (x/y=→"Y_axis":dbl)
            n84 = Bundle By Name(cluster=T4 {"left"=0, "top"=0, "right"=0, "bottom"=0} ("rect"), "left"=w158, "top"=w157, "right"=w164, "bottom"=w163) -> (w156:T4)
            n85 = case shown="False" w201 {
              tunnel: w190 -> [_ w238]
              frame False {
              }
              frame True {
                # "Set Slider Range"
                n86 = call "GetFramesPerSecond.vi"("Camera Handle In"=w238) -> ("FPS"=→"FPS":dbl)  [unwired: 8 in, 2 out]
                n87 = call "GetExposureRange.vi"("Camera Handle In"=w238) -> ("max"=w248:dbl, "min"=w249:dbl, "intervall"=w247:dbl)  [unwired: 6 in, 2 out]
                n88 = Bundle("min"=w249, "max"=w248, "intervall"=w247) -> (w250:cluster{"min":dbl, "max":dbl, "intervall":dbl})  [unwired: 1 in]
                n89 = property on="Exposure time (ms)" class="Schieberegler (strikt)"("Scale.Minimum"=w249, "Scale.Maximum"=w248, "Scale.Increment"=w247) -> ()  [unwired: 2 in, 2 out]
                n90 = property on="Exposure time (ms)" class="Schieberegler (strikt)"("Data Range"=w250) -> ()  [unwired: 2 in, 2 out]
                n91 = call "GetFrameTimeRange.vi"("Camera Handle In"=w238) -> ("max"=w244:dbl, "min"=w243:dbl, "interval"=w240:dbl)  [unwired: 6 in, 2 out]
                n92 = Reciprocal(x=w244) -> (1/x=w242:dbl)
                n93 = Reciprocal(x=w243) -> (1/x=w241:dbl)
                n94 = property on="Frame rate" class="Schieberegler (strikt)"("Minimum"=w242, "Maximum"=w241, "Increment"=w240) -> ()  [unwired: 2 in, 2 out]
                n95 = property on="Frame rate" class="Schieberegler (strikt)"("Scale.Minimum"=w242, "Scale.Maximum"=w241, "Scale.Increment"=w240) -> ()  [unwired: 2 in, 2 out]
                n96 = call "GetPixelClockRange.vi"("Camera Handle In"=w238) -> ("Max"=w246:i32, "Min"=w245:i32)  [unwired: 7 in, 2 out]
                n97 = property on="Pixel clock" class="Schieberegler (strikt)"("Scale.Minimum"=w245, "Scale.Maximum"=w246) -> ()  [unwired: 2 in, 2 out]
                n98 = property on="Pixel clock" class="Schieberegler (strikt)"("Minimum"=w245, "Maximum"=w246) -> ()  [unwired: 2 in, 2 out]
                n99 = call "SetAOI.vi"("Camera Handle In"=w238, "Mode"=32771) -> ("Width Out"=→"Width":i32, "Height Out"=→"Height":i32)  [unwired: 8 in, 4 out]
              }
            }
            n100 = case shown="False" w197 {
              tunnel: w190 -> [_ w207]
              frame False {
              }
              frame True {
                # "Set Exposure time, Pixelclock\nand Framerate"
                n101 = call "ThorSetExposureTime.vi"("Mode"=u16 32900, "Exposure Time"="Exposure time (ms)", "Camera Handle In"=w207) -> ()  [unwired: 6 in, 3 out]
                n102 = call "SetFrameRate.vi"("FPS"="Frame rate", "Camera Handle In"=w207) -> ()  [unwired: 7 in, 3 out]
                n103 = call "SetPixelClock.vi"("Mode"=32770, "Pixel Clock"="Pixel clock", "Camera Handle In"=w207) -> ()  [unwired: 6 in, 3 out]
                n104 = call "SetAutoParameter.vi"("enable"="Autogain", "Param"=34816, "Camera Handle In"=w207) -> ("Camera Handle Out"=w215:u32)  [unwired: 6 in, 2 out]
                n105 = case shown="False" "Autogain" {
                  tunnel: w215 -> [w231 w234]
                  frame False {
                    # "Set Master Gain"
                    n106 = call "SetHardwareGain.vi"("Master Gain"="Master Gain", "Camera Handle In"=w231) -> ()  [unwired: 7 in, 3 out]
                  }
                  frame True {
                    w233 = 32768 items=["IS_GET_MASTER_GAIN"=32768]
                    # "On active AutoGain\nset Master Gain Slider Value"
                    n107 = call "SetHardwareGain.vi"("Mode"=w233, "Camera Handle In"=w234) -> ("Value"=w235:i32)  [unwired: 7 in, 2 out]
                    n108 = property on="Master Gain" class="Slide (strict)"("Value"=w235) -> ()  [unwired: 2 in, 2 out]
                  }
                }
                n109 = case shown="False" "Hotpixel correction 2" {
                  tunnel: w207 -> [w228 w230]
                  frame False {
                    n110 = call "SetHotPixelCorrection.vi"("Mode"=0, "Camera Handle In"=w228) -> ()  [unwired: 7 in, 3 out]
                  }
                  frame True {
                    n111 = call "SetHotPixelCorrection.vi"("Mode"=2, "Camera Handle In"=w230) -> ()  [unwired: 7 in, 3 out]
                  }
                }
                n112 = case shown="True" "Blacklevel compensation" {
                  tunnel: w207 -> [w223 w226]
                  tunnel: "Blacklevel Offset" -> [w221 w224]
                  frame False {
                    n113 = call "SetBlCompensation.vi"("Mode"=0, "offset"=w221, "Camera Handle In"=w223) -> ()  [unwired: 6 in, 3 out]
                  }
                  frame True {
                    n114 = call "SetBlCompensation.vi"("Mode"=1, "offset"=w224, "Camera Handle In"=w226) -> ()  [unwired: 6 in, 3 out]
                  }
                }
                n115 = case shown="True" "Edge Filter Enable / Disable" {
                  tunnel: w207 -> [w217 w220]
                  frame False {
                    n116 = call "SetEdgeEnhancement.vi"("Mode"=0, "Camera Handle In"=w217) -> ()  [unwired: 8 in, 2 out]
                  }
                  frame True {
                    n117 = call "SetEdgeEnhancement.vi"("Mode"="Edge Filter", "Camera Handle In"=w220) -> ()  [unwired: 8 in, 2 out]
                  }
                }
              }
            }
            n118 = local read "Frame rate"() -> (w196:dbl)
            n119 = Reciprocal(x=w196) -> (1/x=w195:dbl)
            n120 = Multiply(x=w195, y=1000) -> (x*y=w193:dbl)
            n121 = Wait Until Next ms Multiple(millisecond multiple=w193) -> ()  [unwired: 1 out]
          }
          event "Reset": Value Change {
            n122 = event-data() -> ()  [unwired: 1 in, 6 out]
            n123 = Unbundle(w284) -> ("Device Z"=w283:refnum<k24>, "Device X"=w282:refnum<k24>, "Device Y"=w281:refnum<k24>)
            n124 = stacked-sequence {
              tunnel: w283 -> [w294 _ _ _ _ w312 w317 w318]
              tunnel: w281 -> [_ _ w298 _ w308 _ _ w319]
              tunnel: w282 -> [_ w295 _ w304 _ _ _ w320]
              frame #0 {
                # "Move Z to maxinum"
                n125 = invoke class="KCubeDCServo" method="MoveTo"(reference=w294, "position"=12.0, "waitTimeout"=0) -> ()  [unwired: 2 in, 5 out]
                n126 = Wait (ms)(milliseconds to wait=u32 10000) -> ()  [unwired: 1 out]
              }
              frame #1 {
                # "Make X home"
                n127 = invoke class="KCubeDCServo" method="Home"(reference=w295, "waitTimeout"=0) -> ()  [unwired: 2 in, 4 out]
                n128 = Wait (ms)(milliseconds to wait=u32 20000) -> ()  [unwired: 1 out]
              }
              frame #2 {
                # "Make Y home"
                n129 = invoke class="KCubeDCServo" method="Home"(reference=w298, "waitTimeout"=0) -> ()  [unwired: 2 in, 4 out]
                n130 = Wait (ms)(milliseconds to wait=u32 20000) -> ()  [unwired: 1 out]
              }
              frame #3 {
                # "Move X to center"
                n131 = invoke class="KCubeDCServo" method="MoveTo"(reference=w304, "position"=7.0, "waitTimeout"=0) -> ()  [unwired: 2 in, 5 out]
                n132 = Wait (ms)(milliseconds to wait=u32 5000) -> ()  [unwired: 1 out]
              }
              frame #4 {
                # "Move Y to center"
                n133 = invoke class="KCubeDCServo" method="MoveTo"(reference=w308, "position"=7.0, "waitTimeout"=0) -> ()  [unwired: 2 in, 5 out]
                n134 = Wait (ms)(milliseconds to wait=u32 5000) -> ()  [unwired: 1 out]
              }
              frame #5 {
                # "Z: home"
                n135 = invoke class="KCubeDCServo" method="Home"(reference=w312, "waitTimeout"=0) -> (reference out=w309:refnum<k24>)  [unwired: 2 in, 3 out]
                n136 = Wait (ms)(milliseconds to wait=u32 20000) -> ()  [unwired: 1 out]
                n137 = invoke class="KCubeDCServo" method="ClearDeviceExceptions"(reference=w309) -> ()  [unwired: 2 in, 3 out]
              }
              frame #6 {
                # "Move satge along Z about 0.5mm"
                n138 = invoke class="KCubeDCServo" method="MoveTo"(reference=w317, "position"=4.5, "waitTimeout"=0) -> (reference out=w313:refnum<k24>)  [unwired: 2 in, 4 out]
                n139 = invoke class="KCubeDCServo" method="ClearDeviceExceptions"(reference=w313) -> ()  [unwired: 2 in, 3 out]
                n140 = Wait (ms)(milliseconds to wait=u32 5000) -> ()  [unwired: 1 out]
              }
              frame #7 {
                n141 = invoke class="KCubeDCServo" method="ClearDeviceExceptions"(reference=w318) -> ()  [unwired: 2 in, 3 out]
                n142 = invoke class="KCubeDCServo" method="ClearDeviceExceptions"(reference=w320) -> ()  [unwired: 2 in, 3 out]
                n143 = invoke class="KCubeDCServo" method="ClearDeviceExceptions"(reference=w319) -> ()  [unwired: 2 in, 3 out]
                n144 = call "Display Message to User"("Enable"=TRUE, "Message"="Reset has been completed!!") -> ()  [unwired: 8 in, 2 out]
              }
            }
          }
          event "Scan": Value Change {
            n145 = event-data() -> ()  [unwired: 1 in, 6 out]
            n146 = Unbundle By Name(w323) -> ("left"=w333:i16, "top"=w331:i16, "right"=w332:i16, "bottom"=w330:i16)
            n147 = stacked-sequence {
              tunnel: w334 -> [_ w370 _ _]
              tunnel: w333 -> [_ w352 w403 _]
              tunnel: w332 -> [_ _ w404 _]
              tunnel: w331 -> [_ w351 w396 _]
              tunnel: w330 -> [_ _ w397 _]
              tunnel: w329 -> [_ w355 w395 _]
              tunnel: w328 -> [_ w354 _ _]
              tunnel: [_ w353 _ _] -> w327
              tunnel: w326 -> [w338 _ w394 _]
              tunnel: w325 -> [w339 _ w393 _]
              tunnel: "Save Path" -> [w341 _ w392 _]
              frame #0 {
                n148 = Unbundle(w339) -> ("Height"=w344:i32, "Width"=w343:i32)
                n149 = Build Path(base path=w341, name or relative path="Crop_Area.png") -> (appended path=w345:path)
                n150 = call "GetActImgMem.vi"("Camera Handle In"=w338) -> ("Image Memory Out"=w348:u8[])  [unwired: 7 in, 3 out]
                n151 = Reshape Array(w348, w344, w343) -> (w349:u8[][])
                n152 = call <vilib>:"Flatten Pixmap.vi"("colors"=u32[] [0, 65793, 131586, 197379, 263172, 328965, 394758, 460551, 526344, 592137, 657930, 723723, 789516, 855309, 921102, 986895, 1052688, 1118481, 1184274, 1250067, 1315860, 1381653, 1447446, 1513239, 1579032, 1644825, 1710618, 1776411, 1842204, 1907997, 1973790, 2039583, 2105376, 2171169, 2236962, 2302755, 2368548, 2434341, 2500134, 2565927, 2631720, 2697513, 2763306, 2829099, 2894892, 2960685, 3026478, 3092271, 3158064, 3223857, 3289650, 3355443, 3421236, 3487029, 3552822, 3618615, 3684408, 3750201, 3815994, 3881787, 3947580, 4013373, 4079166, 4144959, 4210752, 4276545, 4342338, 4408131, 4473924, 4539717, 4605510, 4671303, 4737096, 4802889, 4868682, 4934475, 5000268, 5066061, 5131854, 5197647, 5263440, 5329233, 5395026, 5460819, 5526612, 5592405, 5658198, 5723991, 5789784, 5855577, 5921370, 5987163, 6052956, 6118749, 6184542, 6250335, 6316128, 6381921, 6447714, 6513507, 6579300, 6645093, 6710886, 6776679, 6842472, 6908265, 6974058, 7039851, 7105644, 7171437, 7237230, 7303023, 7368816, 7434609, 7500402, 7566195, 7631988, 7697781, 7763574, 7829367, 7895160, 7960953, 8026746, 8092539, 8158332, 8224125, 8289918, 8355711, 8421504, 8487297, 8553090, 8618883, 8684676, 8750469, 8816262, 8882055, 8947848, 9013641, 9079434, 9145227, 9211020, 9276813, 9342606, 9408399, 9474192, 9539985, 9605778, 9671571, 9737364, 9803157, 9868950, 9934743, 10000536, 10066329, 10132122, 10197915, 10263708, 10329501, 10395294, 10461087, 10526880, 10592673, 10658466, 10724259, 10790052, 10855845, 10921638, 10987431, 11053224, 11119017, 11184810, 11250603, 11316396, 11382189, 11447982, 11513775, 11579568, 11645361, 11711154, 11776947, 11842740, 11908533, 11974326, 12040119, 12105912, 12171705, 12237498, 12303291, 12369084, 12434877, 12500670, 12566463, 12632256, 12698049, 12763842, 12829635, 12895428, 12961221, 13027014, 13092807, 13158600, 13224393, 13290186, 13355979, 13421772, 13487565, 13553358, 13619151, 13684944, 13750737, 13816530, 13882323, 13948116, 14013909, 14079702, 14145495, 14211288, 14277081, 14342874, 14408667, 14474460, 14540253, 14606046, 14671839, 14737632, 14803425, 14869218, 14935011, 15000804, 15066597, 15132390, 15198183, 15263976, 15329769, 15395562, 15461355, 15527148, 15592941, 15658734, 15724527, 15790320, 15856113, 15921906, 15987699, 16053492, 16119285, 16185078, 16250871, 16316664, 16382457, 16448250, 16514043, 16579836, 16645629, 16711422, 0] ("output array 2"), "8-bit pixmap"=w349) -> ("image data"=w346:T16)  [unwired: 9 in]
                n153 = Wait (ms)(milliseconds to wait=u32 300) -> ()  [unwired: 1 out]
                n154 = call <vilib>:"Write PNG File.vi"("image data"=w346, "path to PNG file"=w345) -> ()  [unwired: 8 in, 2 out]
              }
              frame #1 {
                n155 = Unbundle By Name(w370) -> ("Laser X"=w362:dbl, "Laser Y"=w361:dbl)
                n156 = Subtract(x=w362, y=w352) -> (x-y=w360:dbl)
                n157 = Subtract(x=w361, y=w351) -> (x-y=w358:dbl)
                n158 = Divide(x=0.0877, y=1000.0) -> (x/y=w359:dbl)
                n159 = Multiply(x=w359, y=w360) -> (x*y=w357:dbl)
                n160 = Multiply(x=w359, y=w358) -> (x*y=w356:dbl)
                n161 = call "StageReadPos.vi"("error in (no error)"=w354, "Stage Select"=StageSelect."X axis", "Device In"=w355) -> ("error out"=w369:errorcluster, "CurrentPosition"=w367:dbl)  [unwired: 7 in]
                n162 = call "StageReadPos.vi"("error in (no error)"=w354, "Stage Select"=StageSelect."Y axis", "Device In"=w355) -> ("error out"=w365:errorcluster, "CurrentPosition"=w364:dbl)  [unwired: 7 in]
                n163 = stacked-sequence {
                  tunnel: w369 -> [w389 _]
                  tunnel: w367 -> [w387 _]
                  tunnel: [w385 _] -> w363
                  tunnel: w357 -> [w384 _]
                  tunnel: w355 -> [w383 _]
                  frame #0 {
                    n164 = Add(x=w384, y=w387) -> (x+y=w386:dbl)
                    n165 = call "StageToPos.vi"("error in (no error)"=w389, "Move to pos"=w386, "Stage Select"=StageSelect."X axis", "Device In"=w383) -> ("error out"=w385:errorcluster)  [unwired: 7 in]
                  }
                  frame #1 {
                    n166 = Wait (ms)(milliseconds to wait=u32 400) -> ()  [unwired: 1 out]
                  }
                }
                n167 = stacked-sequence {
                  tunnel: w365 -> [w380 _]
                  tunnel: w364 -> [w379 _]
                  tunnel: w363 -> [w377 _]
                  tunnel: w356 -> [w375 _]
                  tunnel: w355 -> [w374 _]
                  tunnel: [w373 _] -> w353
                  frame #0 {
                    n168 = Add(x=w375, y=w379) -> (x+y=w378:dbl)
                    n169 = call "StageToPos.vi"("error in (no error)"=w380, "Move to pos"=w378, "Stage Select"=StageSelect."Y axis", "Device In"=w374) -> ("error out"=w376:errorcluster)  [unwired: 7 in]
                    n170 = Merge Errors(w377, w376) -> (w373:errorcluster)
                  }
                  frame #1 {
                    n171 = Wait (ms)(milliseconds to wait=u32 400) -> ()  [unwired: 1 out]
                  }
                }
                n172 = Wait (ms)(milliseconds to wait=u32 100) -> ()  [unwired: 1 out]
              }
              frame #2 {
                n173 = Subtract(x=w397, y=w396) -> (x-y=w399:i16)
                n174 = Subtract(x=w404, y=w403) -> (x-y=w402:i16)
                n175 = Divide(x=w399, y=i16 50) -> (x/y=w391:dbl)
                n176 = Divide(x=w402, y=i16 50) -> (x/y=w400:dbl)
                n177 = for {
                  N: w391 -> [w411]
                  tunnel: w400 -> [w405]
                  tunnel: w395 -> [w415]
                  tunnel: w394 -> [w414]
                  tunnel: w393 -> [w413]
                  tunnel: w392 -> [w412]
                  i -> [w408]
                  n178 = Round Toward -Infinity(1:w405) -> (0:→"Total_Frame_X":dbl)
                  n179 = Increment(x=w408) -> (x+1=→"Frame_Y":i32)
                  n180 = Divide(x=w408, y=2) -> (x/y=w420:dbl)
                  n181 = Round Toward -Infinity(1:w420) -> (0:w417:dbl)
                  n182 = Round Toward +Infinity(x=w420) -> (ceil(x): smallest int >= x=w418:dbl)
                  n183 = Equal?(x=w418, y=w417) -> (x = y?=w416:bool)
                  n184 = stacked-sequence {
                    tunnel: w416 -> [_ w433 w485]
                    tunnel: w405 -> [_ _ w484]
                    tunnel: w415 -> [w430 _ w483]
                    tunnel: w414 -> [_ w434 w482]
                    tunnel: w413 -> [_ w435 w481]
                    tunnel: w412 -> [_ w436 w480]
                    tunnel: w408 -> [_ w432 w479]
                    tunnel: w405 -> [_ w431 w478]
                    tunnel: [_ _ w477] -> w410
                    frame #0 {
                      w428 = 1 items=["Forward"=1, "Backward"=2] ("direction")
                      n185 = Unbundle By Name(w430) -> ("Device Y"=w429:refnum<k24>)  [unwired: 2 out]
                      n186 = Divide(x=0.0877 ("y"), y=1000.0) -> (x/y=w421:dbl)
                      n187 = Multiply(x=50.0, y=w421) -> (x*y=w424:dbl)
                      n188 = invoke class="KCubeDCServo" method="MoveRelative"(reference=w429, "direction"=w428, "stepSize"=w424, "waitTimeout"=0) -> ()  [unwired: 2 in, 6 out]
                      n189 = Wait (ms)(milliseconds to wait=u32 300) -> ()  [unwired: 1 out]
                    }
                    frame #1 {
                      n190 = case shown="False" w433 {
                        tunnel: w436 -> [w443 w462]
                        tunnel: w435 -> [w441 w461]
                        tunnel: w434 -> [w442 w460]
                        tunnel: w432 -> [w439 w458]
                        tunnel: w431 -> [w438 _]
                        frame False {
                          n191 = Round Toward -Infinity(1:w438) -> (0:w437:dbl)
                          n192 = Increment(x=w439) -> (x+1=w444:i32)
                          n193 = Number To Decimal String(number=w437) -> (decimal integer string=w440:string)  [unwired: 1 in]
                          n194 = Number To Decimal String(number=w444) -> (decimal integer string=w449:string)  [unwired: 1 in]
                          n195 = Concatenate Strings("x" ("string"), w440, "_y" ("string"), w449, ".png" ("string")) -> (w453:string)
                          n196 = Unbundle(w441) -> ("Height"=w447:i32, "Width"=w446:i32)
                          n197 = Build Path(base path=w443, name or relative path=w453) -> (appended path=w448:path)
                          n198 = call "GetActImgMem.vi"("Camera Handle In"=w442) -> ("Image Memory Out"=w456:u8[])  [unwired: 7 in, 3 out]
                          n199 = Reshape Array(w456, w447, w446) -> (w457:u8[][])
                          n200 = call <vilib>:"Flatten Pixmap.vi"("colors"=u32[] [0, 65793, 131586, 197379, 263172, 328965, 394758, 460551, 526344, 592137, 657930, 723723, 789516, 855309, 921102, 986895, 1052688, 1118481, 1184274, 1250067, 1315860, 1381653, 1447446, 1513239, 1579032, 1644825, 1710618, 1776411, 1842204, 1907997, 1973790, 2039583, 2105376, 2171169, 2236962, 2302755, 2368548, 2434341, 2500134, 2565927, 2631720, 2697513, 2763306, 2829099, 2894892, 2960685, 3026478, 3092271, 3158064, 3223857, 3289650, 3355443, 3421236, 3487029, 3552822, 3618615, 3684408, 3750201, 3815994, 3881787, 3947580, 4013373, 4079166, 4144959, 4210752, 4276545, 4342338, 4408131, 4473924, 4539717, 4605510, 4671303, 4737096, 4802889, 4868682, 4934475, 5000268, 5066061, 5131854, 5197647, 5263440, 5329233, 5395026, 5460819, 5526612, 5592405, 5658198, 5723991, 5789784, 5855577, 5921370, 5987163, 6052956, 6118749, 6184542, 6250335, 6316128, 6381921, 6447714, 6513507, 6579300, 6645093, 6710886, 6776679, 6842472, 6908265, 6974058, 7039851, 7105644, 7171437, 7237230, 7303023, 7368816, 7434609, 7500402, 7566195, 7631988, 7697781, 7763574, 7829367, 7895160, 7960953, 8026746, 8092539, 8158332, 8224125, 8289918, 8355711, 8421504, 8487297, 8553090, 8618883, 8684676, 8750469, 8816262, 8882055, 8947848, 9013641, 9079434, 9145227, 9211020, 9276813, 9342606, 9408399, 9474192, 9539985, 9605778, 9671571, 9737364, 9803157, 9868950, 9934743, 10000536, 10066329, 10132122, 10197915, 10263708, 10329501, 10395294, 10461087, 10526880, 10592673, 10658466, 10724259, 10790052, 10855845, 10921638, 10987431, 11053224, 11119017, 11184810, 11250603, 11316396, 11382189, 11447982, 11513775, 11579568, 11645361, 11711154, 11776947, 11842740, 11908533, 11974326, 12040119, 12105912, 12171705, 12237498, 12303291, 12369084, 12434877, 12500670, 12566463, 12632256, 12698049, 12763842, 12829635, 12895428, 12961221, 13027014, 13092807, 13158600, 13224393, 13290186, 13355979, 13421772, 13487565, 13553358, 13619151, 13684944, 13750737, 13816530, 13882323, 13948116, 14013909, 14079702, 14145495, 14211288, 14277081, 14342874, 14408667, 14474460, 14540253, 14606046, 14671839, 14737632, 14803425, 14869218, 14935011, 15000804, 15066597, 15132390, 15198183, 15263976, 15329769, 15395562, 15461355, 15527148, 15592941, 15658734, 15724527, 15790320, 15856113, 15921906, 15987699, 16053492, 16119285, 16185078, 16250871, 16316664, 16382457, 16448250, 16514043, 16579836, 16645629, 16711422, 0] ("output array 2"), "8-bit pixmap"=w457) -> ("image data"=w454:T16)  [unwired: 9 in]
                          n201 = Wait (ms)(milliseconds to wait=u32 300) -> ()  [unwired: 1 out]
                          n202 = call <vilib>:"Write PNG File.vi"("image data"=w454, "path to PNG file"=w448) -> ()  [unwired: 8 in, 2 out]
                        }
                        frame True {
                          n203 = Increment(x=w458) -> (x+1=w463:i32)
                          n204 = Number To Decimal String(number=w463) -> (decimal integer string=w468:string)  [unwired: 1 in]
                          n205 = Concatenate Strings("x" ("string"), "0" ("string"), "_y" ("string"), w468, ".png" ("string")) -> (w472:string)
                          n206 = Unbundle(w461) -> ("Height"=w466:i32, "Width"=w465:i32)
                          n207 = Build Path(base path=w462, name or relative path=w472) -> (appended path=w467:path)
                          n208 = call "GetActImgMem.vi"("Camera Handle In"=w460) -> ("Image Memory Out"=w475:u8[])  [unwired: 7 in, 3 out]
                          n209 = Reshape Array(w475, w466, w465) -> (w476:u8[][])
                          n210 = call <vilib>:"Flatten Pixmap.vi"("colors"=u32[] [0, 65793, 131586, 197379, 263172, 328965, 394758, 460551, 526344, 592137, 657930, 723723, 789516, 855309, 921102, 986895, 1052688, 1118481, 1184274, 1250067, 1315860, 1381653, 1447446, 1513239, 1579032, 1644825, 1710618, 1776411, 1842204, 1907997, 1973790, 2039583, 2105376, 2171169, 2236962, 2302755, 2368548, 2434341, 2500134, 2565927, 2631720, 2697513, 2763306, 2829099, 2894892, 2960685, 3026478, 3092271, 3158064, 3223857, 3289650, 3355443, 3421236, 3487029, 3552822, 3618615, 3684408, 3750201, 3815994, 3881787, 3947580, 4013373, 4079166, 4144959, 4210752, 4276545, 4342338, 4408131, 4473924, 4539717, 4605510, 4671303, 4737096, 4802889, 4868682, 4934475, 5000268, 5066061, 5131854, 5197647, 5263440, 5329233, 5395026, 5460819, 5526612, 5592405, 5658198, 5723991, 5789784, 5855577, 5921370, 5987163, 6052956, 6118749, 6184542, 6250335, 6316128, 6381921, 6447714, 6513507, 6579300, 6645093, 6710886, 6776679, 6842472, 6908265, 6974058, 7039851, 7105644, 7171437, 7237230, 7303023, 7368816, 7434609, 7500402, 7566195, 7631988, 7697781, 7763574, 7829367, 7895160, 7960953, 8026746, 8092539, 8158332, 8224125, 8289918, 8355711, 8421504, 8487297, 8553090, 8618883, 8684676, 8750469, 8816262, 8882055, 8947848, 9013641, 9079434, 9145227, 9211020, 9276813, 9342606, 9408399, 9474192, 9539985, 9605778, 9671571, 9737364, 9803157, 9868950, 9934743, 10000536, 10066329, 10132122, 10197915, 10263708, 10329501, 10395294, 10461087, 10526880, 10592673, 10658466, 10724259, 10790052, 10855845, 10921638, 10987431, 11053224, 11119017, 11184810, 11250603, 11316396, 11382189, 11447982, 11513775, 11579568, 11645361, 11711154, 11776947, 11842740, 11908533, 11974326, 12040119, 12105912, 12171705, 12237498, 12303291, 12369084, 12434877, 12500670, 12566463, 12632256, 12698049, 12763842, 12829635, 12895428, 12961221, 13027014, 13092807, 13158600, 13224393, 13290186, 13355979, 13421772, 13487565, 13553358, 13619151, 13684944, 13750737, 13816530, 13882323, 13948116, 14013909, 14079702, 14145495, 14211288, 14277081, 14342874, 14408667, 14474460, 14540253, 14606046, 14671839, 14737632, 14803425, 14869218, 14935011, 15000804, 15066597, 15132390, 15198183, 15263976, 15329769, 15395562, 15461355, 15527148, 15592941, 15658734, 15724527, 15790320, 15856113, 15921906, 15987699, 16053492, 16119285, 16185078, 16250871, 16316664, 16382457, 16448250, 16514043, 16579836, 16645629, 16711422, 0] ("output array 2"), "8-bit pixmap"=w476) -> ("image data"=w473:T16)  [unwired: 9 in]
                          n211 = Wait (ms)(milliseconds to wait=u32 300) -> ()  [unwired: 1 out]
                          n212 = call <vilib>:"Write PNG File.vi"("image data"=w473, "path to PNG file"=w467) -> ()  [unwired: 8 in, 2 out]
                        }
                      }
                    }
                    frame #2 {
                      n213 = case shown="False" w485 {
                        tunnel: w484 -> [w493 w542]
                        tunnel: w483 -> [w492 w541]
                        tunnel: w482 -> [w490 w540]
                        tunnel: w481 -> [w487 w539]
                        tunnel: w480 -> [w491 w538]
                        tunnel: w479 -> [w489 w537]
                        tunnel: w478 -> [w488 _]
                        tunnel: [w486 w536] -> w477
                        frame False {
                          n214 = for {
                            N: w493 -> [_]
                            tunnel: w492 -> [w500]
                            tunnel: w491 -> [w499]
                            tunnel: w490 -> [w498]
                            tunnel: w489 -> [w497]
                            tunnel: w488 -> [w496]
                            tunnel: w487 -> [w495]
                            tunnel: [w494] -> w486
                            i -> [w494]
                            n215 = stacked-sequence {
                              tunnel: w500 -> [_ w505 _]
                              tunnel: w499 -> [_ _ w524]
                              tunnel: w498 -> [_ _ w523]
                              tunnel: w497 -> [_ _ w518]
                              tunnel: w494 -> [_ _ w516]
                              tunnel: w496 -> [_ _ w515]
                              tunnel: w495 -> [_ _ w522]
                              frame #0 {
                                n216 = Wait (ms)(milliseconds to wait=u32 100) -> ()  [unwired: 1 out]
                              }
                              frame #1 {
                                w511 = 2 items=["Forward"=1, "Backward"=2] ("direction")
                                n217 = Unbundle By Name(w505) -> ("Device X"=w506:refnum<k24>)  [unwired: 2 out]
                                n218 = Divide(x=0.0877 ("y"), y=1000.0) -> (x/y=w503:dbl)
                                n219 = Multiply(x=50.0, y=w503) -> (x*y=w507:dbl)
                                n220 = invoke class="KCubeDCServo" method="MoveRelative"(reference=w506, "direction"=w511, "stepSize"=w507, "waitTimeout"=0) -> ()  [unwired: 2 in, 6 out]
                                n221 = Wait (ms)(milliseconds to wait=u32 450) -> ()  [unwired: 1 out]
                              }
                              frame #2 {
                                n222 = Round Toward -Infinity(1:w515) -> (0:w514:dbl)
                                n223 = Decrement(x=w514) -> (x-1=w513:dbl)
                                n224 = Subtract(x=w513, y=w516) -> (x-y=w512:dbl)
                                n225 = Increment(x=w518) -> (x+1=w517:i32)
                                n226 = Number To Decimal String(number=w512) -> (decimal integer string=w527:string)  [unwired: 1 in]
                                n227 = Number To Decimal String(number=w517) -> (decimal integer string=w526:string)  [unwired: 1 in]
                                n228 = Concatenate Strings("x" ("string"), w527, "_y" ("string"), w526, ".png" ("string")) -> (w531:string)
                                n229 = Unbundle(w522) -> ("Height"=w521:i32, "Width"=w520:i32)
                                n230 = Build Path(base path=w524, name or relative path=w531) -> (appended path=w525:path)
                                n231 = call "GetActImgMem.vi"("Camera Handle In"=w523) -> ("Image Memory Out"=w534:u8[])  [unwired: 7 in, 3 out]
                                n232 = Reshape Array(w534, w521, w520) -> (w535:u8[][])
                                n233 = call <vilib>:"Flatten Pixmap.vi"("colors"=u32[] [0, 65793, 131586, 197379, 263172, 328965, 394758, 460551, 526344, 592137, 657930, 723723, 789516, 855309, 921102, 986895, 1052688, 1118481, 1184274, 1250067, 1315860, 1381653, 1447446, 1513239, 1579032, 1644825, 1710618, 1776411, 1842204, 1907997, 1973790, 2039583, 2105376, 2171169, 2236962, 2302755, 2368548, 2434341, 2500134, 2565927, 2631720, 2697513, 2763306, 2829099, 2894892, 2960685, 3026478, 3092271, 3158064, 3223857, 3289650, 3355443, 3421236, 3487029, 3552822, 3618615, 3684408, 3750201, 3815994, 3881787, 3947580, 4013373, 4079166, 4144959, 4210752, 4276545, 4342338, 4408131, 4473924, 4539717, 4605510, 4671303, 4737096, 4802889, 4868682, 4934475, 5000268, 5066061, 5131854, 5197647, 5263440, 5329233, 5395026, 5460819, 5526612, 5592405, 5658198, 5723991, 5789784, 5855577, 5921370, 5987163, 6052956, 6118749, 6184542, 6250335, 6316128, 6381921, 6447714, 6513507, 6579300, 6645093, 6710886, 6776679, 6842472, 6908265, 6974058, 7039851, 7105644, 7171437, 7237230, 7303023, 7368816, 7434609, 7500402, 7566195, 7631988, 7697781, 7763574, 7829367, 7895160, 7960953, 8026746, 8092539, 8158332, 8224125, 8289918, 8355711, 8421504, 8487297, 8553090, 8618883, 8684676, 8750469, 8816262, 8882055, 8947848, 9013641, 9079434, 9145227, 9211020, 9276813, 9342606, 9408399, 9474192, 9539985, 9605778, 9671571, 9737364, 9803157, 9868950, 9934743, 10000536, 10066329, 10132122, 10197915, 10263708, 10329501, 10395294, 10461087, 10526880, 10592673, 10658466, 10724259, 10790052, 10855845, 10921638, 10987431, 11053224, 11119017, 11184810, 11250603, 11316396, 11382189, 11447982, 11513775, 11579568, 11645361, 11711154, 11776947, 11842740, 11908533, 11974326, 12040119, 12105912, 12171705, 12237498, 12303291, 12369084, 12434877, 12500670, 12566463, 12632256, 12698049, 12763842, 12829635, 12895428, 12961221, 13027014, 13092807, 13158600, 13224393, 13290186, 13355979, 13421772, 13487565, 13553358, 13619151, 13684944, 13750737, 13816530, 13882323, 13948116, 14013909, 14079702, 14145495, 14211288, 14277081, 14342874, 14408667, 14474460, 14540253, 14606046, 14671839, 14737632, 14803425, 14869218, 14935011, 15000804, 15066597, 15132390, 15198183, 15263976, 15329769, 15395562, 15461355, 15527148, 15592941, 15658734, 15724527, 15790320, 15856113, 15921906, 15987699, 16053492, 16119285, 16185078, 16250871, 16316664, 16382457, 16448250, 16514043, 16579836, 16645629, 16711422, 0] ("output array 2"), "8-bit pixmap"=w535) -> ("image data"=w532:T16)  [unwired: 9 in]
                                n234 = Wait (ms)(milliseconds to wait=u32 300) -> ()  [unwired: 1 out]
                                n235 = call <vilib>:"Write PNG File.vi"("image data"=w532, "path to PNG file"=w525) -> ()  [unwired: 8 in, 2 out]
                              }
                            }
                          }
                        }
                        frame True {
                          n236 = for {
                            N: w542 -> [_]
                            tunnel: w541 -> [w548]
                            tunnel: w540 -> [w547]
                            tunnel: w539 -> [w546]
                            tunnel: w538 -> [w545]
                            tunnel: w537 -> [w544]
                            tunnel: [w543] -> w536
                            i -> [w543]
                            n237 = stacked-sequence {
                              tunnel: w548 -> [_ w554 _]
                              tunnel: w547 -> [_ _ w574]
                              tunnel: w546 -> [_ _ w573]
                              tunnel: w545 -> [_ _ w571]
                              tunnel: w543 -> [_ _ w561]
                              tunnel: w544 -> [_ _ w563]
                              frame #0 {
                                n238 = Wait (ms)(milliseconds to wait=u32 100) -> ()  [unwired: 1 out]
                              }
                              frame #1 {
                                w559 = 1 items=["Forward"=1, "Backward"=2] ("direction")
                                n239 = Unbundle By Name(w554) -> ("Device X"=w553:refnum<k24>)  [unwired: 2 out]
                                n240 = Divide(x=0.0877 ("y"), y=1000.0) -> (x/y=w550:dbl)
                                n241 = Multiply(x=50.0, y=w550) -> (x*y=w555:dbl)
                                n242 = invoke class="KCubeDCServo" method="MoveRelative"(reference=w553, "direction"=w559, "stepSize"=w555, "waitTimeout"=0) -> ()  [unwired: 2 in, 6 out]
                                n243 = Wait (ms)(milliseconds to wait=u32 400) -> ()  [unwired: 1 out]
                              }
                              frame #2 {
                                n244 = Increment(x=w561) -> (x+1=w560:i32)
                                n245 = Increment(x=w563) -> (x+1=w562:i32)
                                n246 = Number To Decimal String(number=w562) -> (decimal integer string=w566:string)  [unwired: 1 in]
                                n247 = Number To Decimal String(number=w560) -> (decimal integer string=w567:string)  [unwired: 1 in]
                                n248 = Concatenate Strings("x" ("string"), w567, "_y" ("string"), w566, ".png" ("string")) -> (w572:string)
                                n249 = Build Path(base path=w571, name or relative path=w572) -> (appended path=w565:path)
                                n250 = call "GetActImgMem.vi"("Camera Handle In"=w574) -> ("Image Memory Out"=w577:u8[])  [unwired: 7 in, 3 out]
                                n251 = Unbundle(w573) -> ("Height"=w578:i32, "Width"=w579:i32)
                                n252 = Reshape Array(w577, w578, w579) -> (w580:u8[][])
                                n253 = call <vilib>:"Flatten Pixmap.vi"("colors"=u32[] [0, 65793, 131586, 197379, 263172, 328965, 394758, 460551, 526344, 592137, 657930, 723723, 789516, 855309, 921102, 986895, 1052688, 1118481, 1184274, 1250067, 1315860, 1381653, 1447446, 1513239, 1579032, 1644825, 1710618, 1776411, 1842204, 1907997, 1973790, 2039583, 2105376, 2171169, 2236962, 2302755, 2368548, 2434341, 2500134, 2565927, 2631720, 2697513, 2763306, 2829099, 2894892, 2960685, 3026478, 3092271, 3158064, 3223857, 3289650, 3355443, 3421236, 3487029, 3552822, 3618615, 3684408, 3750201, 3815994, 3881787, 3947580, 4013373, 4079166, 4144959, 4210752, 4276545, 4342338, 4408131, 4473924, 4539717, 4605510, 4671303, 4737096, 4802889, 4868682, 4934475, 5000268, 5066061, 5131854, 5197647, 5263440, 5329233, 5395026, 5460819, 5526612, 5592405, 5658198, 5723991, 5789784, 5855577, 5921370, 5987163, 6052956, 6118749, 6184542, 6250335, 6316128, 6381921, 6447714, 6513507, 6579300, 6645093, 6710886, 6776679, 6842472, 6908265, 6974058, 7039851, 7105644, 7171437, 7237230, 7303023, 7368816, 7434609, 7500402, 7566195, 7631988, 7697781, 7763574, 7829367, 7895160, 7960953, 8026746, 8092539, 8158332, 8224125, 8289918, 8355711, 8421504, 8487297, 8553090, 8618883, 8684676, 8750469, 8816262, 8882055, 8947848, 9013641, 9079434, 9145227, 9211020, 9276813, 9342606, 9408399, 9474192, 9539985, 9605778, 9671571, 9737364, 9803157, 9868950, 9934743, 10000536, 10066329, 10132122, 10197915, 10263708, 10329501, 10395294, 10461087, 10526880, 10592673, 10658466, 10724259, 10790052, 10855845, 10921638, 10987431, 11053224, 11119017, 11184810, 11250603, 11316396, 11382189, 11447982, 11513775, 11579568, 11645361, 11711154, 11776947, 11842740, 11908533, 11974326, 12040119, 12105912, 12171705, 12237498, 12303291, 12369084, 12434877, 12500670, 12566463, 12632256, 12698049, 12763842, 12829635, 12895428, 12961221, 13027014, 13092807, 13158600, 13224393, 13290186, 13355979, 13421772, 13487565, 13553358, 13619151, 13684944, 13750737, 13816530, 13882323, 13948116, 14013909, 14079702, 14145495, 14211288, 14277081, 14342874, 14408667, 14474460, 14540253, 14606046, 14671839, 14737632, 14803425, 14869218, 14935011, 15000804, 15066597, 15132390, 15198183, 15263976, 15329769, 15395562, 15461355, 15527148, 15592941, 15658734, 15724527, 15790320, 15856113, 15921906, 15987699, 16053492, 16119285, 16185078, 16250871, 16316664, 16382457, 16448250, 16514043, 16579836, 16645629, 16711422, 0] ("output array 2"), "8-bit pixmap"=w580) -> ("image data"=w575:T16)  [unwired: 9 in]
                                n254 = call <vilib>:"Write PNG File.vi"("image data"=w575, "path to PNG file"=w565) -> ()  [unwired: 8 in, 2 out]
                                n255 = Wait (ms)(milliseconds to wait=u32 300) -> ()  [unwired: 1 out]
                              }
                            }
                          }
                        }
                      }
                    }
                  }
                  n256 = Increment(x=w410) -> (x+1=→"Frame_X":i32)
                  "Total_Frame_Y" <- w411
                }
              }
              frame #3 {
                n257 = One Button Dialog(message="Scanning is finished!!!", button name ("OK")="OK") -> ()  [unwired: 1 out]
              }
            }
          }
          event "X axis_R": Value Change {
            n258 = event-data() -> ()  [unwired: 1 in, 6 out]
            n259 = Unbundle(w592) -> ("Device X"=w590:refnum<k24>)  [unwired: 2 out]
            n260 = case shown="\"0.05mm\"" w584 {
              tunnel: [0.01 0.1 0.5 1.0 1.5 0.05] -> w583
              frame "0.01mm", Default {
              }
              frame "0.1mm" {
              }
              frame "0.5mm" {
              }
              frame "1mm" {
              }
              frame "1.5mm" {
              }
              frame "0.05mm" {
              }
            }
            n261 = Subtract(x=12.0, y=w583) -> (x-y=w588:dbl)
            n262 = Greater?(x=w588, y=w587) -> (0:w586:bool)
            n263 = case shown="True" w586 {
              tunnel: w590 -> [_ w605]
              tunnel: w583 -> [_ w604]
              frame False {
              }
              frame True {
                w607 = 1 items=["Forward"=1, "Backward"=2] ("direction")
                n264 = invoke class="KCubeDCServo" method="MoveRelative"(reference=w605, "direction"=w607, "stepSize"=w604, "waitTimeout"=0) -> ()  [unwired: 2 in, 6 out]
              }
            }
            n265 = Wait (ms)(milliseconds to wait=u32 50) -> ()  [unwired: 1 out]
          }
          event "X axis_L": Value Change {
            n266 = event-data() -> ()  [unwired: 1 in, 6 out]
            n267 = Unbundle(w614) -> ("Device X"=w613:refnum<k24>)  [unwired: 2 out]
            n268 = case shown="\"0.05mm\"" w609 {
              tunnel: [0.01 0.1 0.5 1.0 1.5 0.05] -> w608
              frame "0.01mm", Default {
              }
              frame "0.1mm" {
              }
              frame "0.5mm" {
              }
              frame "1mm" {
              }
              frame "1.5mm" {
              }
              frame "0.05mm" {
              }
            }
            n269 = Less?(x=w608, y=w612) -> (x < y?=w611:bool)
            n270 = case shown="True" w611 {
              tunnel: w613 -> [_ w628]
              tunnel: w608 -> [_ w627]
              frame False {
              }
              frame True {
                w630 = 2 items=["Forward"=1, "Backward"=2] ("direction")
                n271 = invoke class="KCubeDCServo" method="MoveRelative"(reference=w628, "direction"=w630, "stepSize"=w627, "waitTimeout"=0) -> ()  [unwired: 2 in, 6 out]
              }
            }
            n272 = Wait (ms)(milliseconds to wait=u32 50) -> ()  [unwired: 1 out]
          }
          event "Y axis_B": Value Change {
            n273 = event-data() -> ()  [unwired: 1 in, 6 out]
            n274 = Unbundle(w637) -> ("Device Y"=w636:refnum<k24>)  [unwired: 2 out]
            n275 = case shown="\"0.05mm\"" w632 {
              tunnel: [0.01 0.1 0.5 1.0 1.5 0.05] -> w631
              frame "0.01mm", Default {
              }
              frame "0.1mm" {
              }
              frame "0.5mm" {
              }
              frame "1mm" {
              }
              frame "1.5mm" {
              }
              frame "0.05mm" {
              }
            }
            n276 = Subtract(x=12.0, y=w631) -> (x-y=w638:dbl)
            n277 = Greater?(x=w638, y=w634) -> (0:w635:bool)
            n278 = case shown="True" w635 {
              tunnel: w636 -> [_ w653]
              tunnel: w631 -> [_ w652]
              frame False {
              }
              frame True {
                w655 = 1 items=["Forward"=1, "Backward"=2] ("direction")
                n279 = invoke class="KCubeDCServo" method="MoveRelative"(reference=w653, "direction"=w655, "stepSize"=w652, "waitTimeout"=0) -> ()  [unwired: 2 in, 6 out]
              }
            }
            n280 = Wait (ms)(milliseconds to wait=u32 50) -> ()  [unwired: 1 out]
          }
          event "Y axis_F": Value Change {
            n281 = event-data() -> ()  [unwired: 1 in, 6 out]
            n282 = Unbundle(w661) -> ("Device Y"=w660:refnum<k24>)  [unwired: 2 out]
            n283 = case shown="\"0.05mm\"" w657 {
              tunnel: [0.01 0.1 0.5 1.0 1.5 0.05] -> w656
              frame "0.01mm", Default {
              }
              frame "0.1mm" {
              }
              frame "0.5mm" {
              }
              frame "1mm" {
              }
              frame "1.5mm" {
              }
              frame "0.05mm" {
              }
            }
            n284 = Less?(x=w656, y=w659) -> (x < y?=w662:bool)
            n285 = case shown="True" w662 {
              tunnel: w660 -> [_ w676]
              tunnel: w656 -> [_ w675]
              frame False {
              }
              frame True {
                w678 = 2 items=["Forward"=1, "Backward"=2] ("direction")
                n286 = invoke class="KCubeDCServo" method="MoveRelative"(reference=w676, "direction"=w678, "stepSize"=w675, "waitTimeout"=0) -> ()  [unwired: 2 in, 6 out]
              }
            }
            n287 = Wait (ms)(milliseconds to wait=u32 50) -> ()  [unwired: 1 out]
          }
          event "Z axis_u": Value Change {
            n288 = event-data() -> ()  [unwired: 1 in, 6 out]
            n289 = Unbundle(w684) -> ("Device Z"=w683:refnum<k24>)  [unwired: 2 out]
            n290 = case shown="\"20step\"" w685 {
              tunnel: [1 5 10 30 300 3000] -> w686
              frame "1step", Default {
              }
              frame "2step" {
              }
              frame "5step" {
              }
              frame "10step" {
              }
              frame "15step" {
              }
              frame "20step" {
              }
            }
            n291 = invoke class="KCubeDCServo" method="SetJogStepSize_DeviceUnit"(reference=w683, "stepSize"=w686) -> (reference out=w680:refnum<k24>)  [unwired: 2 in, 3 out]
            n292 = Less?(x=w681, y=11.5) -> (x < y?=w682:bool)
            n293 = case shown="True" w682 {
              tunnel: w680 -> [_ w694]
              frame False {
              }
              frame True {
                w696 = 1 items=["Forward"=1, "Backward"=2] ("direction")
                n294 = invoke class="KCubeDCServo" method="MoveJog"(reference=w694, "direction"=w696, "waitTimeout"=0) -> ()  [unwired: 2 in, 5 out]
              }
            }
            n295 = Wait (ms)(milliseconds to wait=u32 50) -> ()  [unwired: 1 out]
          }
          event "Z axis_d": Value Change {
            n296 = event-data() -> ()  [unwired: 1 in, 6 out]
            n297 = Unbundle(w709) -> ("Device Z"=w710:refnum<k24>)  [unwired: 2 out]
            n298 = case shown="\"20step\"" w708 {
              tunnel: [1 5 10 30 300 3000] -> w711
              frame "1step", Default {
              }
              frame "2step" {
              }
              frame "5step" {
              }
              frame "10step" {
              }
              frame "15step" {
              }
              frame "20step" {
              }
            }
            n299 = invoke class="KCubeDCServo" method="SetJogStepSize_DeviceUnit"(reference=w710, "stepSize"=w711) -> (reference out=w707:refnum<k24>)  [unwired: 2 in, 3 out]
            n300 = Less?(x=0.01 ("y"), y=w705) -> (x < y?=w706:bool)
            n301 = case shown="True" w706 {
              tunnel: w707 -> [_ w718]
              frame False {
              }
              frame True {
                w720 = 2 items=["Forward"=1, "Backward"=2] ("direction")
                n302 = invoke class="KCubeDCServo" method="MoveJog"(reference=w718, "direction"=w720, "waitTimeout"=0) -> ()  [unwired: 2 in, 5 out]
              }
            }
            n303 = Wait (ms)(milliseconds to wait=u32 50) -> ()  [unwired: 1 out]
          }
          event "MoveTo": Value Change {
            n304 = event-data() -> ()  [unwired: 1 in, 6 out]
            n305 = Unbundle(w728) -> ("Device Z"=w727:refnum<k24>)  [unwired: 2 out]
            n306 = invoke class="KCubeDCServo" method="MoveTo"(reference=w727, "position"="Destination", "waitTimeout"=0) -> ()  [unwired: 2 in, 5 out]
            n307 = Wait (ms)(milliseconds to wait=u32 1000) -> ()  [unwired: 1 out]
          }
          event "Snap": Value Change {
            n308 = event-data() -> ()  [unwired: 1 in, 6 out]
            n309 = call "GetActImgMem.vi"("Camera Handle In"=w747) -> ("Image Memory Out"=w742:u8[])  [unwired: 7 in, 3 out]
            n310 = Unbundle(w740) -> ("Height"=w743:i32, "Width"=w744:i32)
            n311 = Reshape Array(w742, w743, w744) -> (w745:u8[][])
            n312 = call <vilib>:"Flatten Pixmap.vi"("colors"=u32[] [0, 65793, 131586, 197379, 263172, 328965, 394758, 460551, 526344, 592137, 657930, 723723, 789516, 855309, 921102, 986895, 1052688, 1118481, 1184274, 1250067, 1315860, 1381653, 1447446, 1513239, 1579032, 1644825, 1710618, 1776411, 1842204, 1907997, 1973790, 2039583, 2105376, 2171169, 2236962, 2302755, 2368548, 2434341, 2500134, 2565927, 2631720, 2697513, 2763306, 2829099, 2894892, 2960685, 3026478, 3092271, 3158064, 3223857, 3289650, 3355443, 3421236, 3487029, 3552822, 3618615, 3684408, 3750201, 3815994, 3881787, 3947580, 4013373, 4079166, 4144959, 4210752, 4276545, 4342338, 4408131, 4473924, 4539717, 4605510, 4671303, 4737096, 4802889, 4868682, 4934475, 5000268, 5066061, 5131854, 5197647, 5263440, 5329233, 5395026, 5460819, 5526612, 5592405, 5658198, 5723991, 5789784, 5855577, 5921370, 5987163, 6052956, 6118749, 6184542, 6250335, 6316128, 6381921, 6447714, 6513507, 6579300, 6645093, 6710886, 6776679, 6842472, 6908265, 6974058, 7039851, 7105644, 7171437, 7237230, 7303023, 7368816, 7434609, 7500402, 7566195, 7631988, 7697781, 7763574, 7829367, 7895160, 7960953, 8026746, 8092539, 8158332, 8224125, 8289918, 8355711, 8421504, 8487297, 8553090, 8618883, 8684676, 8750469, 8816262, 8882055, 8947848, 9013641, 9079434, 9145227, 9211020, 9276813, 9342606, 9408399, 9474192, 9539985, 9605778, 9671571, 9737364, 9803157, 9868950, 9934743, 10000536, 10066329, 10132122, 10197915, 10263708, 10329501, 10395294, 10461087, 10526880, 10592673, 10658466, 10724259, 10790052, 10855845, 10921638, 10987431, 11053224, 11119017, 11184810, 11250603, 11316396, 11382189, 11447982, 11513775, 11579568, 11645361, 11711154, 11776947, 11842740, 11908533, 11974326, 12040119, 12105912, 12171705, 12237498, 12303291, 12369084, 12434877, 12500670, 12566463, 12632256, 12698049, 12763842, 12829635, 12895428, 12961221, 13027014, 13092807, 13158600, 13224393, 13290186, 13355979, 13421772, 13487565, 13553358, 13619151, 13684944, 13750737, 13816530, 13882323, 13948116, 14013909, 14079702, 14145495, 14211288, 14277081, 14342874, 14408667, 14474460, 14540253, 14606046, 14671839, 14737632, 14803425, 14869218, 14935011, 15000804, 15066597, 15132390, 15198183, 15263976, 15329769, 15395562, 15461355, 15527148, 15592941, 15658734, 15724527, 15790320, 15856113, 15921906, 15987699, 16053492, 16119285, 16185078, 16250871, 16316664, 16382457, 16448250, 16514043, 16579836, 16645629, 16711422, 0] ("output array 2"), "8-bit pixmap"=w745) -> ("image data"=w739:T16)  [unwired: 9 in]
            n313 = call <vilib>:"Write PNG File.vi"("image data"=w739) -> ()  [unwired: 9 in, 2 out]
          }
          event "Next step": Value Change {
            n314 = event-data() -> ()  [unwired: 1 in, 6 out]
          }
          event "Live video": Mouse Down {
            # "When the mouse is inside the video area, after the mouse is down and hold, the coordinate of the ROI upper left corner is stored."
            n315 = event-data() -> ("Coords"=w762:T5)  [unwired: 1 in, 7 out]
          }
          event "Live video": Mouse Up {
            # "When the mouse is inside the video area, after the mouse is up, the edge of the ROI is calculated."
            n316 = event-data() -> ("Coords"=w771:T5)  [unwired: 1 in, 7 out]
            n317 = property on="Live video" class="Pict"() -> ("Position"=w769:T17)  [unwired: 2 in, 2 out]
            n318 = Unbundle By Name "Start"(w770) -> ("Horizontal"=w791:i32, "Vertical"=w788:i32)
            n319 = Unbundle By Name(w771) -> ("Horizontal"=w785:i32, "Vertical"=w782:i32)
            n320 = Unbundle By Name(w769) -> ("Left"=w793:i32, "Top"=w792:i32)
            n321 = Subtract(x=w791, y=3) -> (x-y=w789:i32)
            n322 = Subtract(x=w788, y=3) -> (x-y=w787:i32)
            n323 = Subtract(x=w785, y=3) -> (x-y=w783:i32)
            n324 = Subtract(x=w782, y=3) -> (x-y=w780:i32)
            n325 = Subtract(x=w789, y=w793) -> (x-y=w779:i32)
            n326 = Subtract(x=w787, y=w792) -> (x-y=w778:i32)
            n327 = Subtract(x=w783, y=w793) -> (x-y=w765:i32)
            n328 = Subtract(x=w780, y=w792) -> (x-y=w764:i32)
            n329 = Divide(x=w779, y=w772) -> (x/y=w777:dbl)
            n330 = Divide(x=w778, y=w772) -> (x/y=w776:dbl)
            n331 = Divide(x=w765, y=w772) -> (x/y=w775:dbl)
            n332 = Divide(x=w764, y=w772) -> (x/y=w774:dbl)
            n333 = Bundle By Name(cluster=T4 {"left"=0, "top"=0, "right"=0, "bottom"=0} ("rect"), "left"=w777, "top"=w776, "right"=w775, "bottom"=w774) -> (w773:T4)
          }
          event "Quit": Value Change {
            # "Add recover initial position\nZ: max\nX: middle\nY: middle\nand also need to attch a limit"
            # "When user clicks the STOP button, program will jump to \"Shut down\" state"
            n334 = event-data() -> ()  [unwired: 1 in, 6 out]
          }
          event "Focus": Value Change {
            # "When clicking the Focus button, following steps will be executed: \n1. move the stage to 4 different Z positions and take an image at each position;\n2. crop the image to get 4 ROIs and use them to find the focal plane;\n3. move the stage to the focal plane."
            n335 = event-data() -> ()  [unwired: 1 in, 6 out]
            n336 = Divide(x="Jog size (um)", y=1000.0) -> (x/y=w804:dbl)
            n337 = Divide(x=w804, y=2.0) -> (x/y=w806:dbl)
            n338 = call "StageReadPos.vi"("error in (no error)"=w847, "Stage Select"=StageSelect."Z axis", "Device In"=w818) -> ("error out"=w845:errorcluster, "CurrentPosition"=w811:dbl)  [unwired: 7 in]
            n339 = Unbundle By Name(w840) -> ("Device Z"=w837:refnum<k24>)
            n340 = Add(x=w811, y=w804) -> (x+y=w809:dbl)
            n341 = Subtract(x=w811, y=w804) -> (x-y=w841:dbl)
            n342 = invoke class="KCubeDCServo" method="GetVelocityParams"(reference=w837) -> ("GetVelocityParams"=w836:refnum<k24>)  [unwired: 2 in, 2 out]
            n343 = Subtract(x=w811, y=w806) -> (x-y=w812:dbl)
            n344 = Subtract(x=w809, y=w806) -> (x-y=w810:dbl)
            n345 = Add(x=w810, y=w804) -> (x+y=w807:dbl)
            n346 = Subtract(x=w841, y=w806) -> (x-y=w805:dbl)
            n347 = Subtract(x=w807, y=w806) -> (x-y=w808:dbl)
            n348 = Build Array(w805, w812, w810, w808) -> (w838:dbl[])
            n349 = property class="VelocityParameters"(reference=w836) -> (reference out=w834:refnum<k24>, error out=w835:errorcluster, "Acceleration"=w833:dbl)  [unwired: 1 in]
            n350 = property class="VelocityParameters"(reference=w834, error in=w835) -> ("MaxVelocity"=w832:dbl)  [unwired: 2 out]
            n351 = for {
              tunnel: w838 -> [w876] mode=indexing
              tunnel: w845 -> [w879]
              tunnel: w818 -> [w878]
              tunnel: [w869] -> w839
              tunnel: w844 -> [w872]
              tunnel: w843 -> [w871]
              tunnel: [w851] -> w827 mode=indexing
              tunnel: w842 -> [w867]
              tunnel: w804 -> [w865]
              tunnel: w833 -> [w856]
              tunnel: w832 -> [w855]
              w859 = 0.9 ("y")
              n352 = call "StageToPos.vi"("error in (no error)"=w879, "Move to pos"=w876, "Stage Select"=StageSelect."Z axis", "Device In"=w878) -> ("error out"=w864:errorcluster)  [unwired: 7 in]
              n353 = call "MovingTime.vi"("error in"=w864, "Acc (mm/s^2)"=w856, "MaxV (mm/s)"=w855, "Distance (mm)"=w865) -> ("error out"=w863:errorcluster, "time (s)"=w862:dbl)  [unwired: 6 in]
              n354 = Multiply(x=w862, y=2.0) -> (x*y=w858:dbl)
              n355 = Greater?(x=w858, y=w859) -> (0:w860:bool)
              n356 = Select(t=w858, s=w860, f=w859) -> (s? t:f=w857:dbl)
              "Delay (s)" <- w857
              n357 = call "Time Delay"("error in (no error)"=w863, "Delay Time (s)"=w857) -> ("error out"=w866:errorcluster)  [unwired: 9 in]
              n358 = call "GetActImgMem.vi"("error in"=w866, "Camera Handle In"=w872) -> ("error out"=w870:errorcluster, "Image Memory Out"=w873:u8[])  [unwired: 6 in, 2 out]
              n359 = Unbundle(w871) -> ("Height"=w874:i32, "Width"=w875:i32)
              n360 = Reshape Array(w873, w874, w875) -> (w850:u8[][])
              n361 = call <vilib>:"Flatten Pixmap.vi"("colors"=u32[] [0, 65793, 131586, 197379, 263172, 328965, 394758, 460551, 526344, 592137, 657930, 723723, 789516, 855309, 921102, 986895, 1052688, 1118481, 1184274, 1250067, 1315860, 1381653, 1447446, 1513239, 1579032, 1644825, 1710618, 1776411, 1842204, 1907997, 1973790, 2039583, 2105376, 2171169, 2236962, 2302755, 2368548, 2434341, 2500134, 2565927, 2631720, 2697513, 2763306, 2829099, 2894892, 2960685, 3026478, 3092271, 3158064, 3223857, 3289650, 3355443, 3421236, 3487029, 3552822, 3618615, 3684408, 3750201, 3815994, 3881787, 3947580, 4013373, 4079166, 4144959, 4210752, 4276545, 4342338, 4408131, 4473924, 4539717, 4605510, 4671303, 4737096, 4802889, 4868682, 4934475, 5000268, 5066061, 5131854, 5197647, 5263440, 5329233, 5395026, 5460819, 5526612, 5592405, 5658198, 5723991, 5789784, 5855577, 5921370, 5987163, 6052956, 6118749, 6184542, 6250335, 6316128, 6381921, 6447714, 6513507, 6579300, 6645093, 6710886, 6776679, 6842472, 6908265, 6974058, 7039851, 7105644, 7171437, 7237230, 7303023, 7368816, 7434609, 7500402, 7566195, 7631988, 7697781, 7763574, 7829367, 7895160, 7960953, 8026746, 8092539, 8158332, 8224125, 8289918, 8355711, 8421504, 8487297, 8553090, 8618883, 8684676, 8750469, 8816262, 8882055, 8947848, 9013641, 9079434, 9145227, 9211020, 9276813, 9342606, 9408399, 9474192, 9539985, 9605778, 9671571, 9737364, 9803157, 9868950, 9934743, 10000536, 10066329, 10132122, 10197915, 10263708, 10329501, 10395294, 10461087, 10526880, 10592673, 10658466, 10724259, 10790052, 10855845, 10921638, 10987431, 11053224, 11119017, 11184810, 11250603, 11316396, 11382189, 11447982, 11513775, 11579568, 11645361, 11711154, 11776947, 11842740, 11908533, 11974326, 12040119, 12105912, 12171705, 12237498, 12303291, 12369084, 12434877, 12500670, 12566463, 12632256, 12698049, 12763842, 12829635, 12895428, 12961221, 13027014, 13092807, 13158600, 13224393, 13290186, 13355979, 13421772, 13487565, 13553358, 13619151, 13684944, 13750737, 13816530, 13882323, 13948116, 14013909, 14079702, 14145495, 14211288, 14277081, 14342874, 14408667, 14474460, 14540253, 14606046, 14671839, 14737632, 14803425, 14869218, 14935011, 15000804, 15066597, 15132390, 15198183, 15263976, 15329769, 15395562, 15461355, 15527148, 15592941, 15658734, 15724527, 15790320, 15856113, 15921906, 15987699, 16053492, 16119285, 16185078, 16250871, 16316664, 16382457, 16448250, 16514043, 16579836, 16645629, 16711422, 0] ("output array 2"), "8-bit pixmap"=w850) -> ("image data"=w854:T16)  [unwired: 9 in]
              n362 = call <vilib>:"Draw Flattened Pixmap.vi"("image data"=w854) -> ("new picture"=w852:picture)  [unwired: 8 in]
              n363 = local write "Live video"(w852) -> ()
              n364 = call "ROI_crop.vi"("error constant"=w870, "roiEdge"=w867, "InputImage"=w850) -> ("error constant 2"=w869:errorcluster, "ROI"=w868:dbl[][])  [unwired: 7 in]
              n365 = To Unsigned Byte Integer(number=w868) -> (unsigned 8bit integer=w851:u8[][])
            }
            n366 = Index Array(array=w827, index (dim 0)=0 ("index (page)")) -> (element=w825:u8[][])  [unwired: 2 in]
            n367 = Index Array(array=w827, index (dim 0)=1 ("index (page)")) -> (element=w824:u8[][])  [unwired: 2 in]
            n368 = Index Array(array=w827, index (dim 0)=2 ("index (page)")) -> (element=w823:u8[][])  [unwired: 2 in]
            n369 = Index Array(array=w827, index (dim 0)=3 ("index (page)")) -> (element=w822:u8[][])  [unwired: 2 in]
            n370 = Bundle By Name(cluster=T13 {"Image2"=[], "Image3"=[], "Image4"=[], "Image1"=[]} ("Imput images"), "Image1"=w825, "Image2"=w824, "Image3"=w823, "Image4"=w822) -> (w821:T13)
            n371 = call "Find_Focus.vi"("error in (no error)"=w839, "Input_Z"=w838, "Imput images"=w821) -> ("error out"=w820:errorcluster, "BestPosition"=w816:dbl)  [unwired: 7 in]
            "Focal plane (mm)" <- w816
            n372 = call "StageToPos.vi"("error in (no error)"=w820, "Move to pos"=w816, "Stage Select"=StageSelect."Z axis", "Device In"=w818) -> ("error out"=w819:errorcluster)  [unwired: 7 in]
          }
          event "Aim": Value Change {
            # "First, you need to draw an ROI, and then when you click the Aim button, the center of the\nview will move to the center of the selected ROI."
            n373 = event-data() -> ()  [unwired: 1 in, 6 out]
            n374 = Unbundle By Name(w916) -> ("left"=w914:i16, "right"=w915:i16, "top"=w909:i16, "bottom"=w908:i16)
            n375 = Unbundle By Name(w882) -> ("Laser X"=w881:dbl, "Laser Y"=w880:dbl)
            n376 = Add(x=w914, y=w915) -> (x+y=w913:i16)
            n377 = Add(x=w909, y=w908) -> (x+y=w910:i16)
            n378 = Divide(x=w913, y=i16 2) -> (x/y=w907:dbl)
            n379 = Divide(x=w910, y=i16 2) -> (x/y=w906:dbl)
            n380 = Subtract(x=w907, y=w881) -> (x-y=w896:dbl)
            n381 = Subtract(x=w906, y=w880) -> (x-y=w901:dbl)
            n382 = Divide(x="Pixel Size Y (um)", y=1000.0) -> (x/y=w897:dbl)
            n383 = Divide(x="Pixel Size X (um)", y=1000.0) -> (x/y=w895:dbl)
            n384 = Multiply(x=w895, y=w896) -> (x*y=w902:dbl)
            n385 = Multiply(x=w901, y=w897) -> (x*y=w900:dbl)
            n386 = call "StageReadPos.vi"("error in (no error)"=w917, "Stage Select"=StageSelect."X axis", "Device In"=w905) -> ("error out"=w894:errorcluster, "CurrentPosition"=w891:dbl)  [unwired: 7 in]
            n387 = call "StageReadPos.vi"("error in (no error)"=w917, "Stage Select"=StageSelect."Y axis", "Device In"=w905) -> ("error out"=w887:errorcluster, "CurrentPosition"=w886:dbl)  [unwired: 7 in]
            n388 = Add(x=w900, y=w886) -> (x+y=w885:dbl)
            n389 = Add(x=w902, y=w891) -> (x+y=w890:dbl)
            n390 = call "StageToPos.vi"("error in (no error)"=w894, "Move to pos"=w890, "Stage Select"=StageSelect."X axis", "Device In"=w905) -> ("error out"=w884:errorcluster)  [unwired: 7 in]
            n391 = call "StageToPos.vi"("error in (no error)"=w887, "Move to pos"=w885, "Stage Select"=StageSelect."Y axis", "Device In"=w905) -> ("error out"=w883:errorcluster)  [unwired: 7 in]
            n392 = Merge Errors(w884, w883) -> (w918:errorcluster)
          }
          event "LaserSpot": Value Change {
            # "First, you need to draw an ROI, and then when you click the Here's Laser button, the center of the\nROI will be stored for Aim use."
            n393 = event-data() -> ()  [unwired: 1 in, 6 out]
            n394 = Unbundle By Name(w927) -> ("left"=w934:i16, "right"=w935:i16, "top"=w929:i16, "bottom"=w928:i16)
            n395 = Add(x=w934, y=w935) -> (x+y=w933:i16)
            n396 = Add(x=w929, y=w928) -> (x+y=w930:i16)
            n397 = Divide(x=w933, y=i16 2) -> (x/y=w923:dbl)
            n398 = Divide(x=w930, y=i16 2) -> (x/y=w922:dbl)
            n399 = Bundle By Name(cluster=T3 {"Laser X"=0.0, "Laser Y"=0.0} ("LaserSpot"), "Laser X"=w923, "Laser Y"=w922) -> (w925:T3)
            n400 = local write "Spot Y"(w922) -> ()
            n401 = local write "Spot X"(w923) -> ()
            "Boolean" <- TRUE ("Boolean")
          }
          event "Left": Value Change {
            n402 = event-data() -> ()  [unwired: 1 in, 6 out]
            n403 = Unbundle By Name(w943) -> ("Laser X"=w941:dbl, "Laser Y"=w942:dbl)
            n404 = Decrement(x=w941) -> (x-1=w940:dbl)
            n405 = Bundle By Name(cluster=T3 {"Laser X"=0.0, "Laser Y"=0.0} ("LaserSpot"), "Laser X"=w940, "Laser Y"=w942) -> (w944:T3)
            n406 = local write "Spot X"(w940) -> ()
          }
          event "Right": Value Change {
            n407 = event-data() -> ()  [unwired: 1 in, 6 out]
            n408 = Unbundle By Name(w954) -> ("Laser X"=w952:dbl, "Laser Y"=w955:dbl)
            n409 = Increment(x=w952) -> (x+1=w951:dbl)
            n410 = Bundle By Name(cluster=T3 {"Laser X"=0.0, "Laser Y"=0.0} ("LaserSpot"), "Laser X"=w951, "Laser Y"=w955) -> (w953:T3)
            n411 = local write "Spot X"(w951) -> ()
          }
          event "Top": Value Change {
            n412 = event-data() -> ()  [unwired: 1 in, 6 out]
            n413 = Unbundle By Name(w966) -> ("Laser X"=w964:dbl, "Laser Y"=w963:dbl)
            n414 = Decrement(x=w963) -> (x-1=w962:dbl)
            n415 = Bundle By Name(cluster=T3 {"Laser X"=0.0, "Laser Y"=0.0} ("LaserSpot"), "Laser X"=w964, "Laser Y"=w962) -> (w965:T3)
            n416 = local write "Spot Y"(w962) -> ()
          }
          event "Down": Value Change {
            n417 = event-data() -> ()  [unwired: 1 in, 6 out]
            n418 = Unbundle By Name(w977) -> ("Laser X"=w975:dbl, "Laser Y"=w974:dbl)
            n419 = Increment(x=w974) -> (x+1=w973:dbl)
            n420 = Bundle By Name(cluster=T3 {"Laser X"=0.0, "Laser Y"=0.0} ("LaserSpot"), "Laser X"=w975, "Laser Y"=w973) -> (w976:T3)
            n421 = local write "Spot Y"(w973) -> ()
          }
          event "Galvo DC": Value Change {
            w985 = T9."Enabled" ("Disabled")
            n422 = event-data() -> ()  [unwired: 1 in, 6 out]
            n423 = call <vilib>:"DAQmx Start Task.vi"("task/channels in"=w989, "error in"=w988) -> ("task out"=w990:refnum<k21>, "error out"=w987:errorcluster)  [unwired: 12 in]
            n424 = property on="Galvo Stop" class="Bool"("DisabledEnum"=w985) -> ()  [unwired: 2 in, 2 out]
            n425 = property on="Galvo Reset" class="Bool"("DisabledEnum"=w985) -> ()  [unwired: 2 in, 2 out]
            n426 = property on="Galvo DC" class="Bool"("DisabledEnum"=T9."Disabled and Grayed Out" ("Disabled")) -> ()  [unwired: 2 in, 2 out]
          }
          event "Galvo Reset": Value Change {
            n427 = event-data() -> ()  [unwired: 1 in, 6 out]
            n428 = local read "a2"() -> (w994:dbl)
            n429 = local read "a0"() -> (w998:dbl)
            n430 = local read "a1"() -> (w997:dbl)
            n431 = call "bo3"("Offset"=w994) -> ("DC"=w999:dynamicdata)  [unwired: 13 in, 1 out]
            n432 = call "bo2"("Offset"=w997) -> ("DC"=w1000:dynamicdata)  [unwired: 13 in, 1 out]
            n433 = call "bo"("Offset"=w998) -> ("DC"=w1001:dynamicdata)  [unwired: 13 in, 1 out]
            n434 = Build Array(w1001, w1000, w999) -> (w996:dynamicdata[])
            n435 = local write "Waveform Graph"(w996) -> ()
            n436 = call "Galvo_Reset.vi"("error in"=w1003, "auto start"=TRUE, "Signal array"=w996, "task/channels in"=w1005) -> ("error out"=w1002:errorcluster, "task out"=w1004:refnum<k21>)  [unwired: 6 in]
          }
          event "Galvo Stop": Value Change {
            n437 = event-data() -> ()  [unwired: 1 in, 6 out]
            n438 = call <vilib>:"DAQmx Stop Task.vi"("task/channels in"=w1015, "error in"=w1013) -> ("task out"=w1012:refnum<k21>, "error out"=w1014:errorcluster)  [unwired: 12 in]
            n439 = property on="Galvo DC" class="Bool"("DisabledEnum"=T9."Enabled" ("Disabled")) -> ()  [unwired: 2 in, 2 out]
            n440 = property on="Galvo Reset" class="Bool"("DisabledEnum"=T9."Disabled and Grayed Out" ("Disabled")) -> ()  [unwired: 2 in, 2 out]
          }
        }
      }
    }
  }
  n441 = call <vilib>:"Simple Error Handler.vi"("error in (no error)"=w10) -> ()  [unwired: 4 in, 5 out]
